vi "transfer char run_subvi_7_24_12a_PD.vi"(0 "VISA session":refnum<visa-resource-name>="GPIB0::17::INSTR", 5 "Var1 sweep settings":T4={"start"=40.0, "stop"=-40.0, "step (linear only)"=-1.0, "sweep spacing (linear: 0)"=0, "sweep mode"=FALSE, "compliance (V)"=100.0, "compliance (A)"=0.001} {"compliance (A)" format="%^.2e"; "compliance (V)" format="%.2f"; "sweep spacing (linear: 0)" items=["linear", "log 10", "log 25", "log 50"]; "step (linear only)" format="%.2f"; "stop" format="%.2f"; "start" format="%.2f"}, 7 "Var2 step settings":T3={"compliance (A)"=0.001, "compliance (V)"=100.0, "start"=-2.0, "total points"=2, "step"=-38.0} {"step" format="%.2f"; "start" format="%.2f"; "compliance (V)" format="%.2f"; "compliance (A)" format="%^.2e"}, 9 "integration time":u32(slide) scale=0.0..2.0, 11 "Input Path":path, 13 "Sample Properties:":T1 {"Date Created" format="%<%x>T"}) -> (1 "Trap Density-STS":dbl, 3 "Trap Density-VT":dbl, 4 "Mobility":dbl, 6 "graphic display":cluster{"trace":dbl[], "trace":dbl[]}(graph), 8 "On/Off Current":dbl, 10 "XY Graph":cluster{dbl[], "trace":dbl[]}[](graph), 12 "Vt":dbl, 14 "STS":dbl, 15 "error?":errorcluster)   [LabVIEW 2011]
uses:
  <vilib>/Utility/file.llb/Write To Spreadsheet File (DBL).vi
  <vilib>/Utility/file.llb/Read From Spreadsheet File (string).vi
  <vilib>/Utility/file.llb/Write To Spreadsheet File (string).vi
  <vilib>/Analysis/NI_AALPro.lvlib
panel:
  out "Array":string[][](array[string])
  in  "Output Path":path
  in  "Temp (K)":dbl=0.001 format="%^.2e"
  in  "NumPts":dbl=5.0
  out "Numeric":dbl
  out "Max R":i32[](listbox)
  out "min r":dbl
  out "max r":dbl
  out "error? 2":errorcluster
  in  "MAXIMUM":ext format="%.2e"
  in  "MINIMUM":ext=-1e-05 format="%_2e"
  out "graphic display 2":cluster{"trace":dbl[], "trace":dbl[]}(graph)
  in  "Y1 axis":string="Id"
  in  "Y2 axis settings":T2 {"MAXIMUM" format="%.9f"; "MINIMUM" format="%.9f"}
  in  "wait time parameter":dbl=1.0
  in  "Value (Either V or A) 4":dbl
  in  "Value (Either V or A) 3":dbl
  in  "Value (Either V or A) 2":dbl
  in  "Value (V or A)":dbl
  in  "compliance (A)":dbl=0.001 format="%^.2e"
  in  "compliance (V)":dbl=100.0 format="%^.2e"
  in  "Iname":string="Is"
  in  "Vname":string="Vs"
  in  "Function":u16(ring)=4 items=["disabled", "Var1", "Var2", "Var1'", "Constant"]
  in  "Mode":u16(ring)=4 items=["V", "I", "VPulse", "IPulse", "Common"]
  in  "Iname 4":string="I4"
  in  "Vname 4":string="V4"
  in  "Function 4":u16(ring)=4 items=["disabled", "Var1", "Var2", "Var1'", "Constant"]
  in  "Mode 4":u16(ring) items=["V", "I", "VPulse", "IPulse", "Common"]
  in  "Iname 3":string="Ig"
  in  "Vname 3":string="Vg"
  in  "Function 3":u16(ring)=1 items=["disabled", "Var1", "Var2", "Var1'", "Constant"]
  in  "Mode 3":u16(ring) items=["V", "I", "VPulse", "IPulse", "Common"]
  in  "Iname 2":string="Id"
  in  "Vname 2":string="Vd"
  in  "Function 2":u16(ring)=2 items=["disabled", "Var1", "Var2", "Var1'", "Constant"]
  in  "Mode 2":u16(ring) items=["V", "I", "VPulse", "IPulse", "Common"]
  in  "reset":bool=TRUE
  # "SMU1"
  # "SMU2"
  # "SMU3"
  # "SMU4"
  # "Sample Properties:"
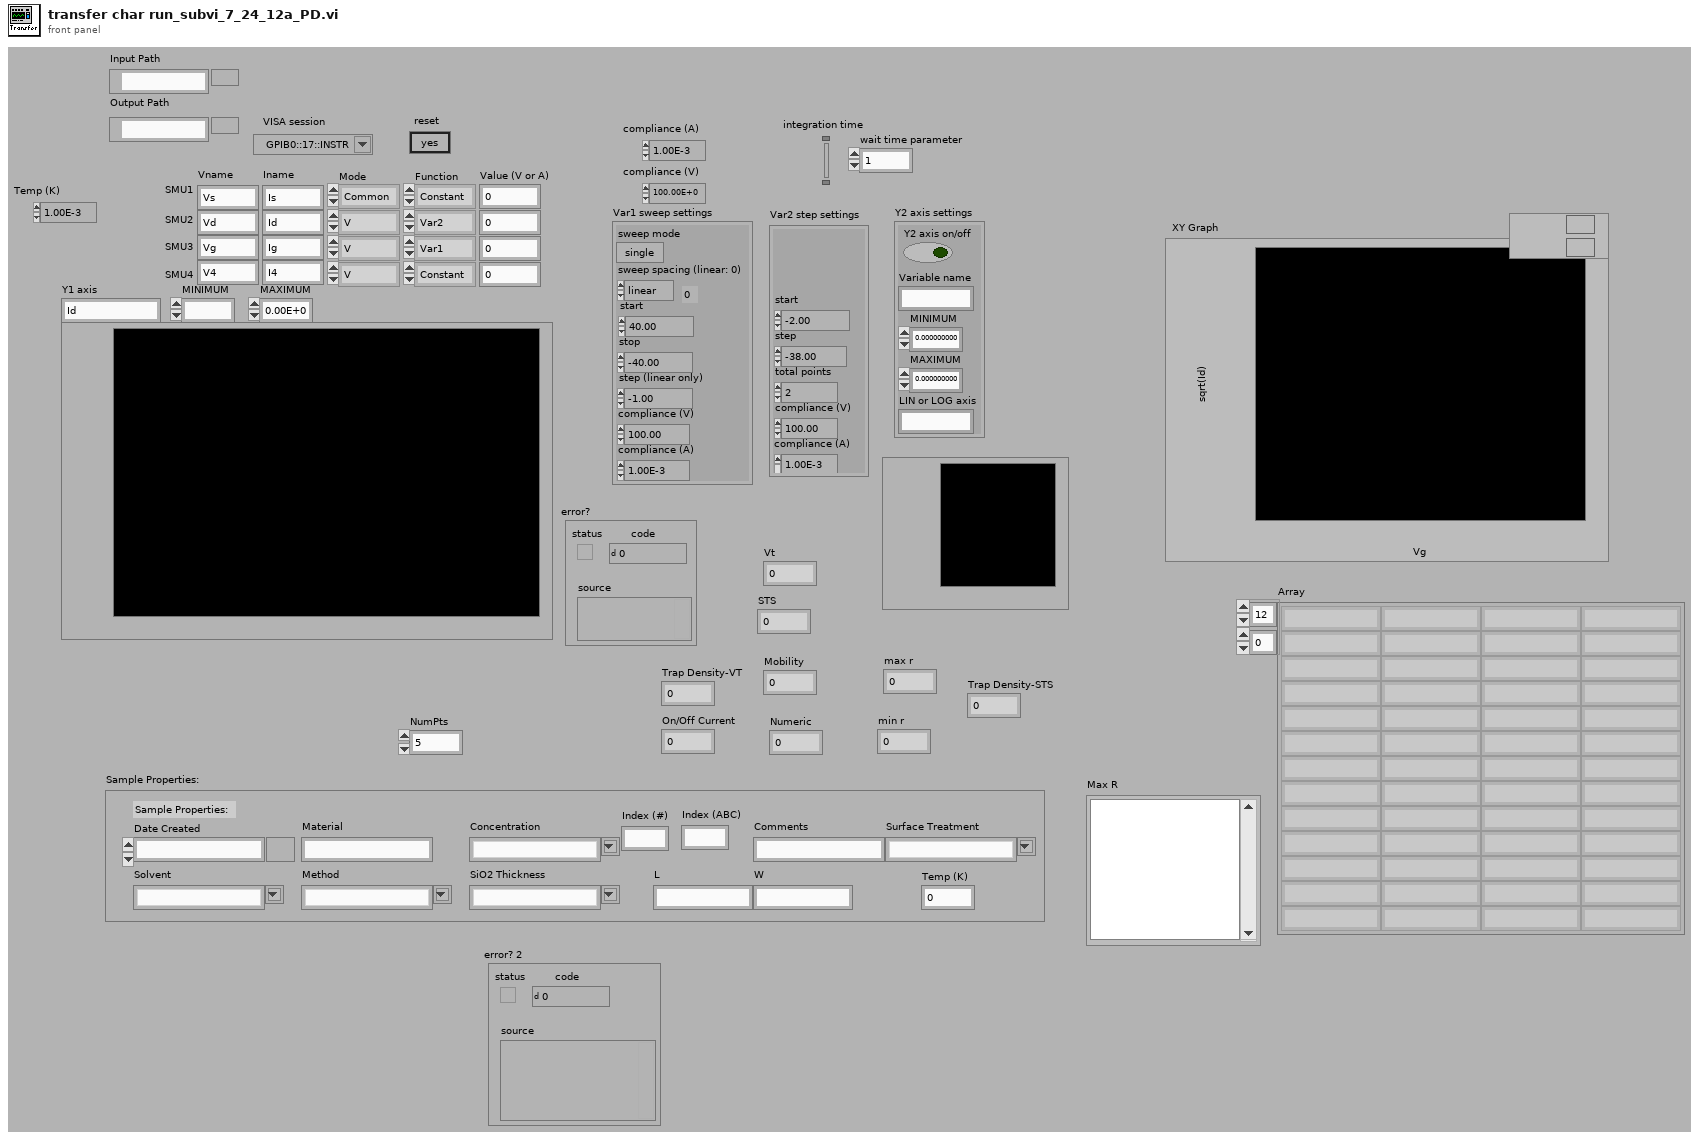
[diagram p1: front panel]
types:
  T1 = cluster{"Date Created":timestamp, "Material":string, "Solvent":string, "Concentration":string, "Method":string, "SiO2 Thickness":string, "Index (#)":string, "Index (ABC)":string, "L":string, "W":string, "Surface Treatment":string, "Comments":string, "Temp (K)":dbl}
  T2 = cluster{"Y2 axis on/off":bool, "MINIMUM":ext, "MAXIMUM":ext, "Variable name":string, "LIN or LOG axis":string}
  T3 = cluster{"compliance (A)":dbl, "compliance (V)":dbl, "start":dbl, "total points":u16, "step":dbl}
  T4 = cluster{"start":dbl, "stop":dbl, "step (linear only)":dbl, "sweep spacing (linear: 0)":u16, "sweep mode":bool, "compliance (V)":dbl, "compliance (A)":dbl}
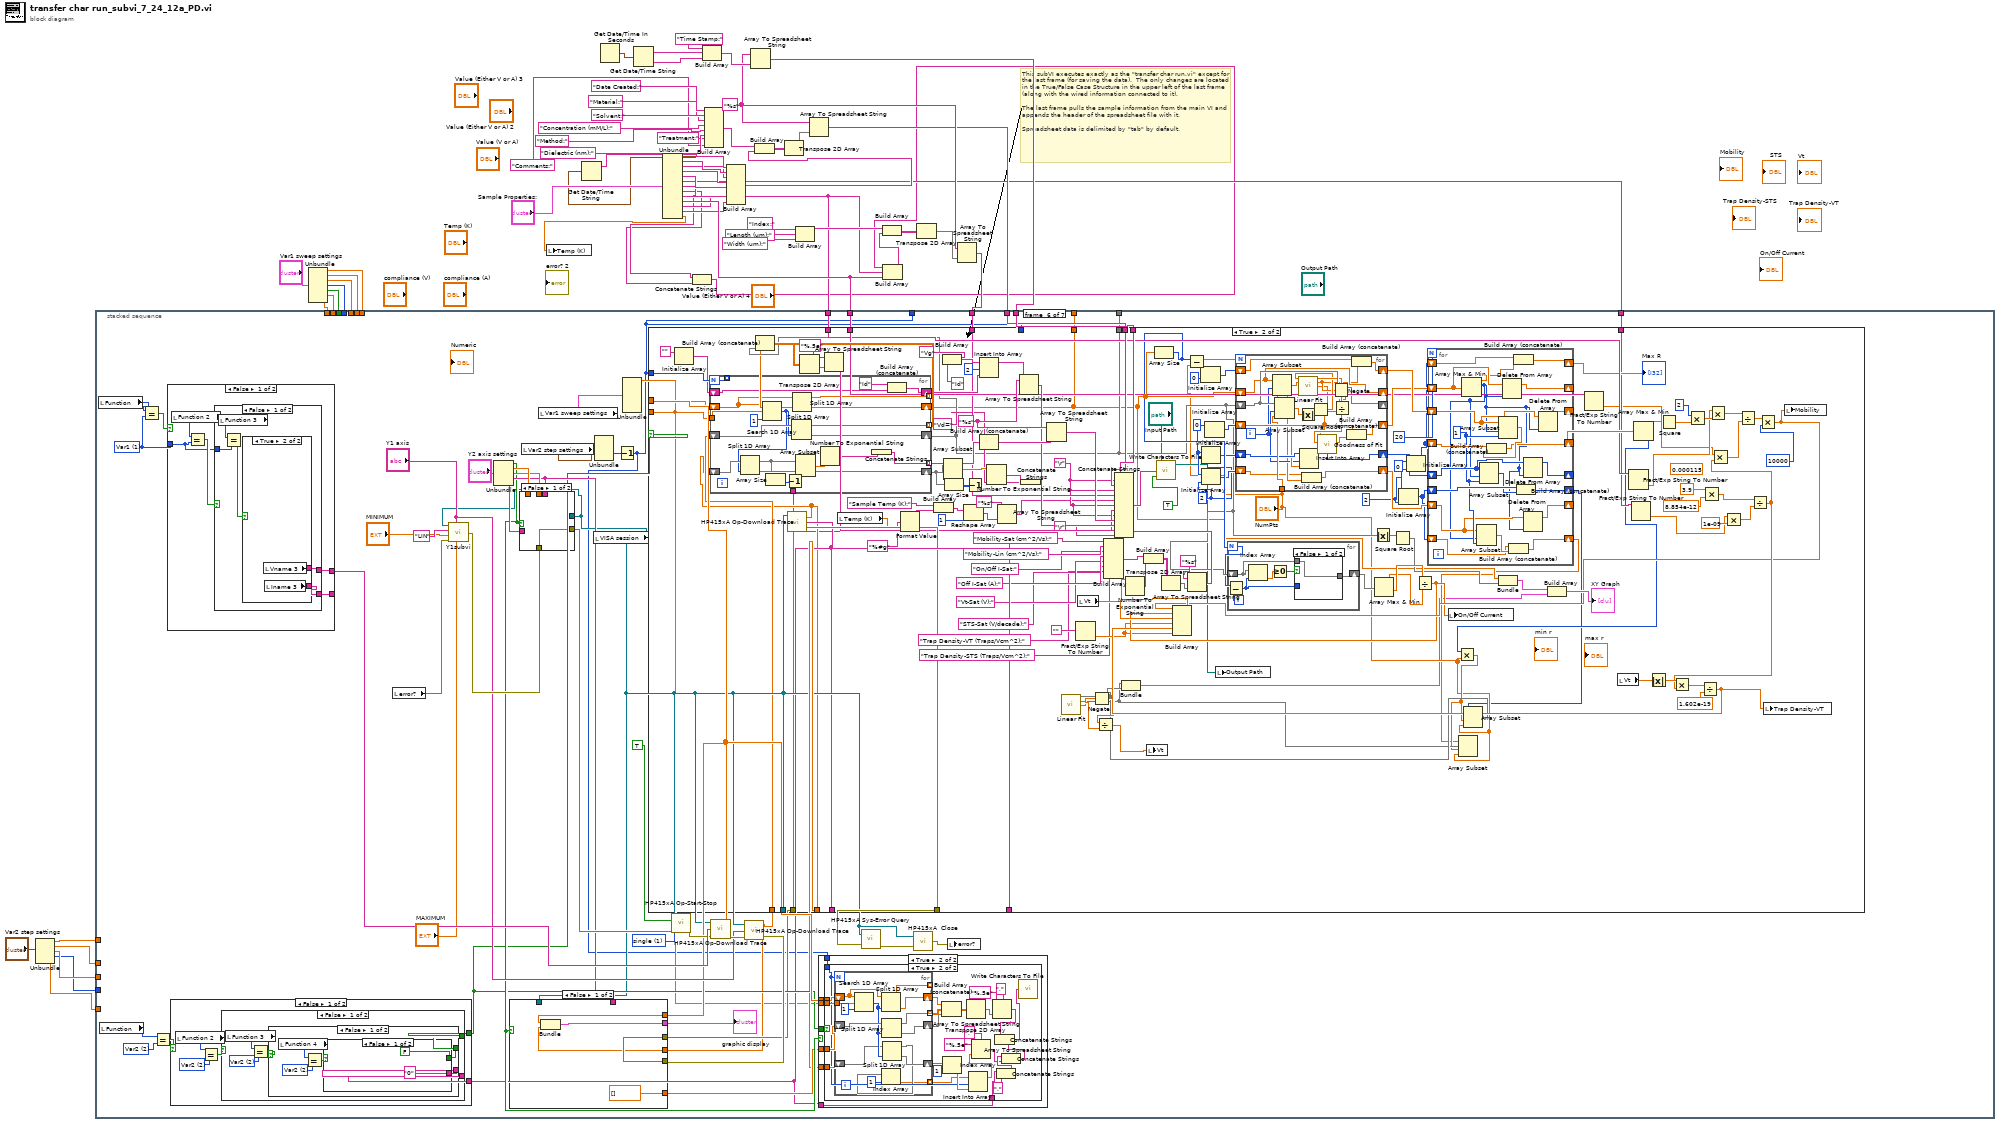
[diagram p0: block diagram]
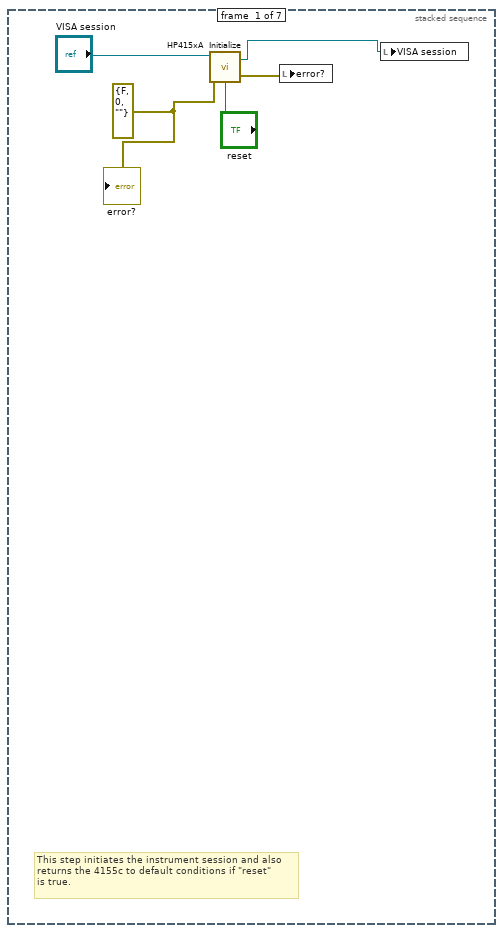
[diagram p2: hidden frame]
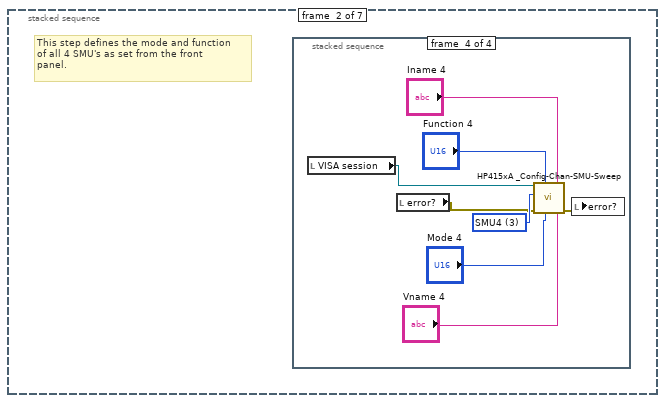
[diagram p3: hidden frame]
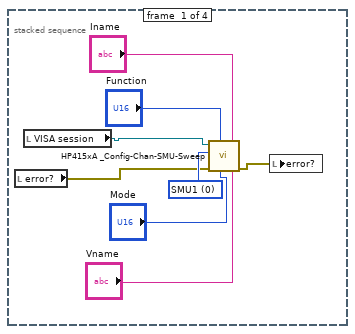
[diagram p4: hidden frame]
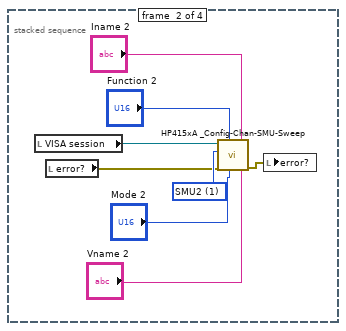
[diagram p5: hidden frame]
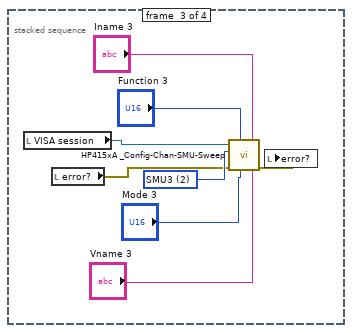
[diagram p6: hidden frame]
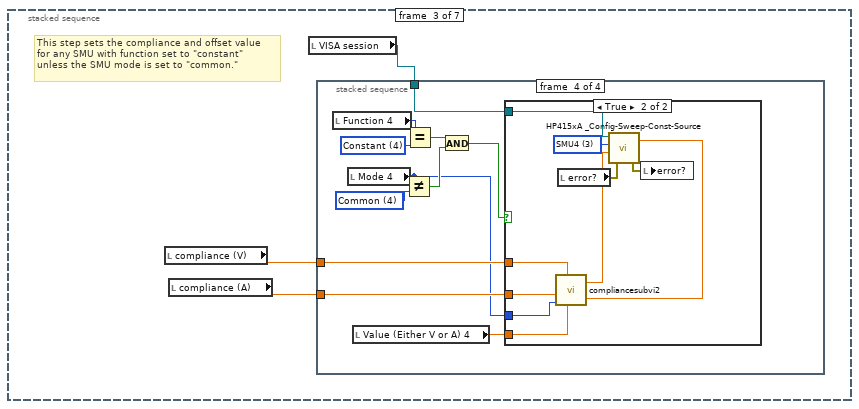
[diagram p7: hidden frame]
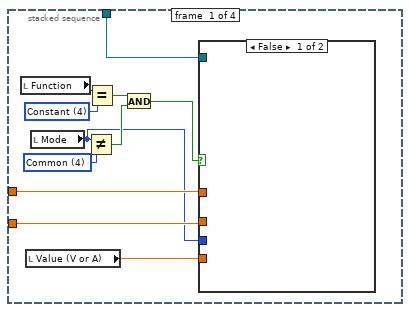
[diagram p8: hidden frame]
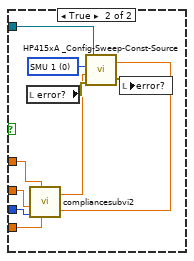
[diagram p9: hidden frame]
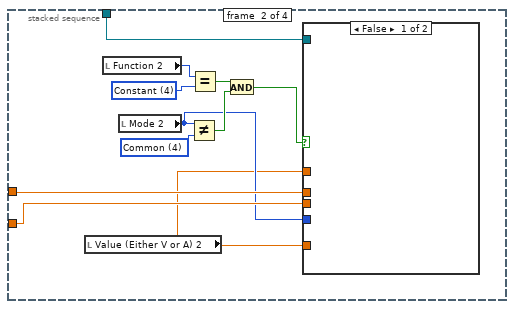
[diagram p10: hidden frame]
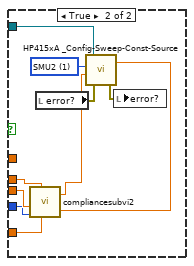
[diagram p11: hidden frame]
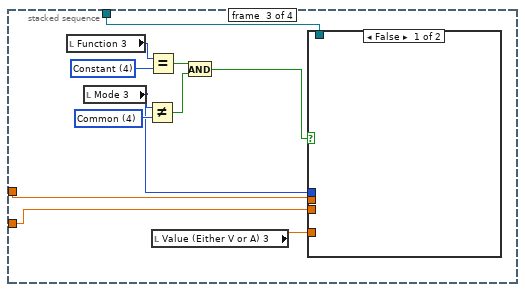
[diagram p12: hidden frame]
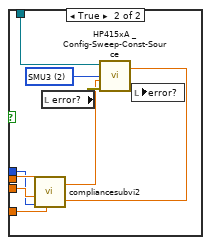
[diagram p13: hidden frame]
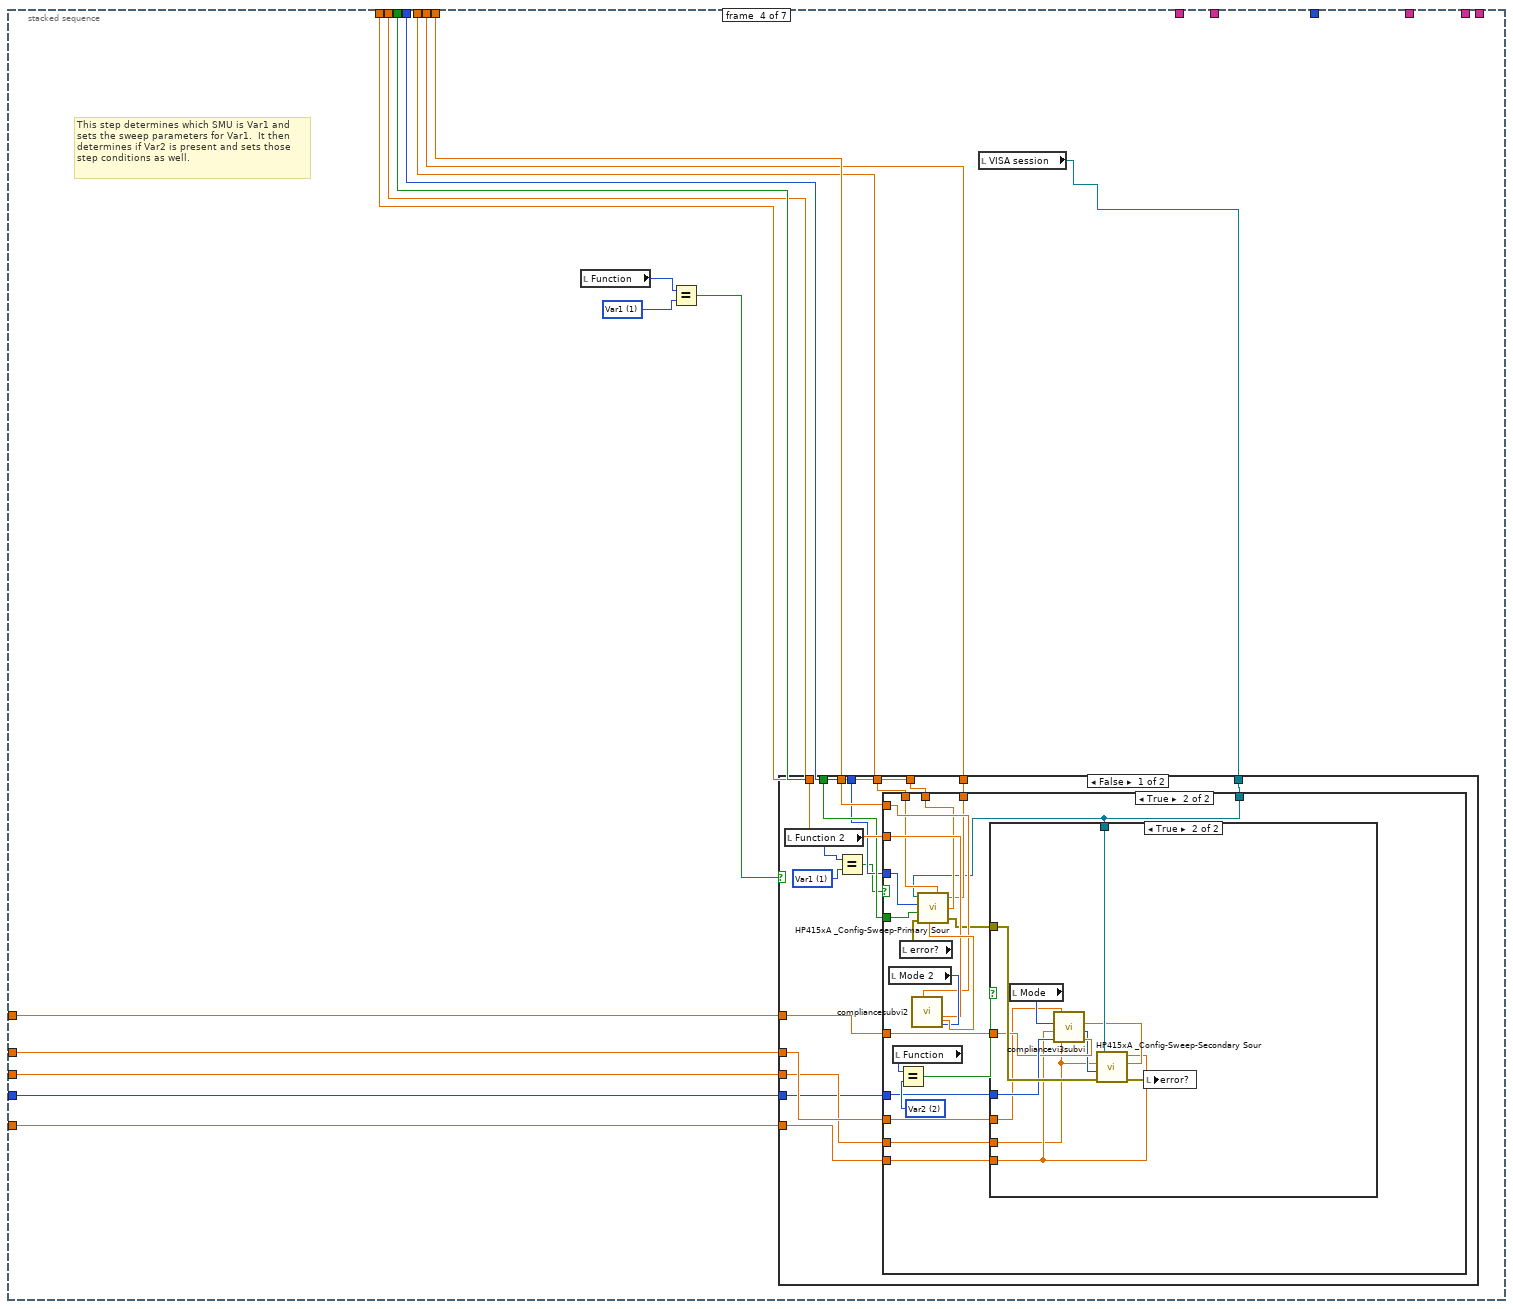
[diagram p15: hidden frame]
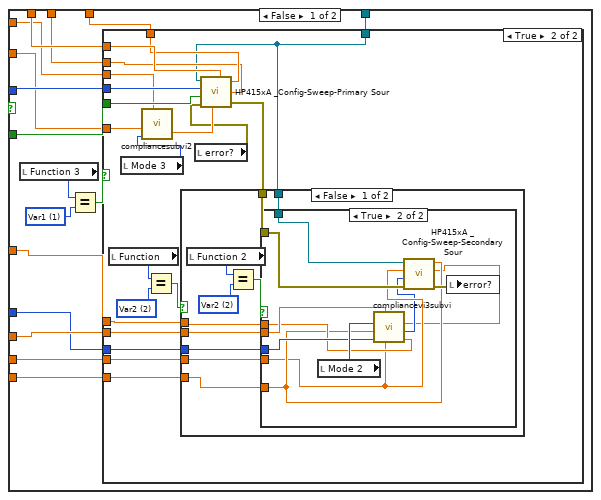
[diagram p16: hidden frame]
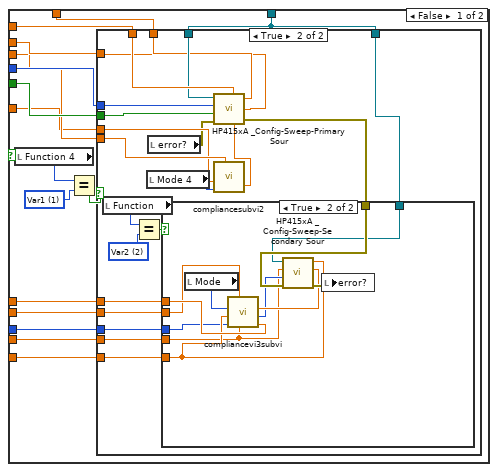
[diagram p17: hidden frame]
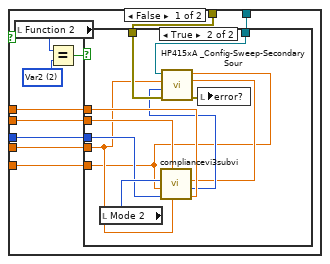
[diagram p19: hidden frame]
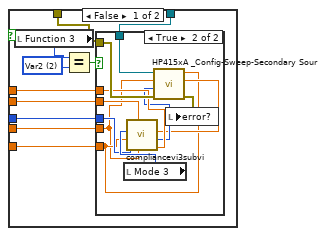
[diagram p20: hidden frame]
diagram:
  w31 = "%s"
  # "This subVI executes exactly as the \"transfer char run.vi\" except for the last frame (for saving the data).  The only changes are located in the True/False Case Structure in the upper left of the last frame (along with the wired information connected to it). \n\nThe last frame pulls the sample information from the main VI and appends the header of the spreadsheet file with it.\n\nSpreadsheet data is delimited by \"tab\" by default."
  n1 = Unbundle("Var2 step settings") -> ("compliance (A)"=w49:dbl, "compliance (V)"=w48:dbl, "start"=w47:dbl, "total points"=w46:u16, "step"=w45:dbl)
  n2 = Unbundle("Var1 sweep settings") -> ("start"=w57:dbl, "stop"=w56:dbl, "step (linear only)"=w55:dbl, "sweep spacing (linear: 0)"=w54:u16, "sweep mode"=w53:bool, "compliance (V)"=w52:dbl, "compliance (A)"=w51:dbl)
  n3 = Get Date/Time In Seconds() -> (seconds since 1Jan1904=w38:timestamp)
  n4 = Get Date/Time String(seconds (now)=w38) -> (date string=w37:string, time string=w36:string)  [unwired: 2 in]
  n5 = Unbundle("Sample Properties:") -> ("Date Created"=w16:timestamp, "Material"=w15:string, "Solvent"=w11:string, "Concentration"=w10:string, "Method"=w14:string, "SiO2 Thickness"=w9:string, "Index (#)"=w4:string, "Index (ABC)"=w3:string, "L"=w7:string, "W"=w8:string, "Surface Treatment"=w6:string, "Comments"=w5:string, "Temp (K)"=w1:dbl)
  n6 = local write "Temp (K)"(w1) -> ()
  n7 = Get Date/Time String(seconds (now)=w16) -> (date string=w43:string)  [unwired: 2 in, 1 out]
  n8 = Concatenate Strings(w4, w3) -> (w2:string)
  n9 = Build Array("Time Stamp:", w37, w36) -> (w35:string[])
  n10 = Build Array("Date Created:", "Material:", "Solvent:", "Concentration (mM/L):", "Method:", "Dielectric (nm):", "Treatment:", "Comments:") -> (w26:string[])
  n11 = Build Array(w43, w15, w11, w10, w14, w9, w6, w5) -> (w25:string[])
  n12 = Array To Spreadsheet String(array=w35, 3:w31) -> (spreadsheet string=w27:string)  [unwired: 1 in]
  n13 = Build Array(w26, w25) -> (w24:string[][])
  n14 = Transpose 2D Array(2D array=w24) -> (transposed array=w23:string[][])
  n15 = Build Array("Index:", "Length (um):", "Width (um):") -> (w22:string[])
  n16 = Array To Spreadsheet String(array=w23, 3:w31) -> (spreadsheet string=w30:string)  [unwired: 1 in]
  n17 = Build Array(w2, w7, w8) -> (w21:string[])
  n18 = Build Array(w22, w21) -> (w20:string[][])
  n19 = Transpose 2D Array(2D array=w20) -> (transposed array=w19:string[][])
  n20 = Array To Spreadsheet String(array=w19, 3:w31) -> (spreadsheet string=w18:string)  [unwired: 1 in]
  n21 = stacked-sequence {
    tunnel: w57 -> [_ _ _ w194 _ _ _]
    tunnel: w56 -> [_ _ _ w193 _ _ _]
    tunnel: w55 -> [_ _ _ w192 _ _ _]
    tunnel: w54 -> [_ _ _ w191 _ _ _]
    tunnel: w53 -> [_ _ _ w190 _ _ _]
    tunnel: w52 -> [_ _ _ w189 _ _ _]
    tunnel: w51 -> [_ _ _ w188 _ _ _]
    tunnel: w49 -> [_ _ _ w187 _ _ _]
    tunnel: w48 -> [_ _ _ w186 _ _ _]
    tunnel: w47 -> [_ _ _ w185 _ _ _]
    tunnel: w46 -> [_ _ _ w184 _ _ _]
    tunnel: w45 -> [_ _ _ w183 _ _ _]
    tunnel: w27 -> [_ _ _ _ _ w557 _]
    tunnel: w30 -> [_ _ _ _ _ w556 _]
    tunnel: w18 -> [_ _ _ _ _ w555 _]
    tunnel: [_ _ _ _ _ w554 _] -> _
    tunnel: [_ _ _ _ _ w553 _] -> _
    tunnel: [_ _ _ _ _ w550 _] -> _
    tunnel: w8 -> [_ _ _ _ _ w552 _]
    tunnel: w7 -> [_ _ _ _ _ w551 _]
    tunnel: w9 -> [_ _ _ _ _ w549 _]
    frame #0 {
      w62 = errorcluster {"status"=FALSE, "code"=0, "source"=""} ("error out")
      # "This step initiates the instrument session and also\nreturns the 4155c to default conditions if \"reset\"\nis true."
      n22 = call "HP415xA  Initialize.vi"("instrument descriptor"="VISA session", "reset"="reset", "error in (no error)"=w62) -> ("VISA session"=w59:refnum<visa-resource-name>, "error out"=w61:errorcluster)  [unwired: 2 in]
      n23 = local write "error?"(w61) -> ()
      n24 = local write "VISA session"(w59) -> ()
      "error?" <- w62
    }
    frame #1 {
      # "This step defines the mode and function\nof all 4 SMU's as set from the front\npanel."
      n25 = stacked-sequence {
        frame #0 {
          w71 = u32 0 items=["SMU1  ", "SMU2  ", "SMU3  ", "SMU4  ", "SMU5  ", "SMU6  "] ("unit to configure")
          n26 = local read "error?"() -> (w66:errorcluster)
          n27 = local read "VISA session"() -> (w64:refnum<visa-resource-name>)
          n28 = call "HP415xA _Config-Chan-SMU-Sweep.vi"("V name (max 6 chars)"="Vname", "I name (max 6 chars)"="Iname", "mode"="Mode", "function"="Function", "error in (no error)"=w66, "unit to configure"=w71, "VISA session"=w64) -> ("error out"=w65:errorcluster)  [unwired: 2 in]
          n29 = local write "error?"(w65) -> ()
        }
        frame #1 {
          w75 = u32 1 items=["SMU1  ", "SMU2  ", "SMU3  ", "SMU4  ", "SMU5  ", "SMU6  "] ("unit to configure")
          n30 = local read "VISA session"() -> (w72:refnum<visa-resource-name>)
          n31 = local read "error?"() -> (w73:errorcluster)
          n32 = call "HP415xA _Config-Chan-SMU-Sweep.vi"("V name (max 6 chars)"="Vname 2", "I name (max 6 chars)"="Iname 2", "mode"="Mode 2", "function"="Function 2", "error in (no error)"=w73, "unit to configure"=w75, "VISA session"=w72) -> ("error out"=w74:errorcluster)  [unwired: 2 in]
          n33 = local write "error?"(w74) -> ()
        }
        frame #2 {
          w83 = u32 2 items=["SMU1  ", "SMU2  ", "SMU3  ", "SMU4  ", "SMU5  ", "SMU6  "] ("unit to configure")
          n34 = local read "VISA session"() -> (w80:refnum<visa-resource-name>)
          n35 = local read "error?"() -> (w81:errorcluster)
          n36 = call "HP415xA _Config-Chan-SMU-Sweep.vi"("V name (max 6 chars)"="Vname 3", "I name (max 6 chars)"="Iname 3", "mode"="Mode 3", "function"="Function 3", "error in (no error)"=w81, "unit to configure"=w83, "VISA session"=w80) -> ("error out"=w82:errorcluster)  [unwired: 2 in]
          n37 = local write "error?"(w82) -> ()
        }
        frame #3 {
          w91 = u32 3 items=["SMU1  ", "SMU2  ", "SMU3  ", "SMU4  ", "SMU5  ", "SMU6  "] ("unit to configure")
          n38 = local read "VISA session"() -> (w88:refnum<visa-resource-name>)
          n39 = local read "error?"() -> (w90:errorcluster)
          n40 = call "HP415xA _Config-Chan-SMU-Sweep.vi"("V name (max 6 chars)"="Vname 4", "I name (max 6 chars)"="Iname 4", "mode"="Mode 4", "function"="Function 4", "error in (no error)"=w90, "unit to configure"=w91, "VISA session"=w88) -> ("error out"=w89:errorcluster)  [unwired: 2 in]
          n41 = local write "error?"(w89) -> ()
        }
      }
    }
    frame #2 {
      # "This step sets the compliance and offset value\nfor any SMU with function set to \"constant\"\nunless the SMU mode is set to \"common.\""
      n42 = local read "compliance (V)"() -> (w97:dbl)
      n43 = local read "compliance (A)"() -> (w98:dbl)
      n44 = local read "VISA session"() -> (w96:refnum<visa-resource-name>)
      n45 = stacked-sequence {
        tunnel: w96 -> [w107 w127 w146 w166]
        tunnel: w98 -> [w101 w123 w144 w164]
        tunnel: w97 -> [w100 w122 w143 w165]
        frame #0 {
          w105 = u16 4 items=["V", "I", "VPulse", "IPulse", "Common"] ("Mode")
          w109 = u16 4 items=["disabled", "Var1", "Var2", "Var1'", "Constant"] ("Function")
          n46 = local read "Function"() -> (w108:u16)
          n47 = local read "Value (V or A)"() -> (w102:dbl)
          n48 = local read "Mode"() -> (w99:u16)
          n49 = Not Equal?(x=w99, y=w105) -> (x != y?=w104:bool)
          n50 = Equal?(x=w108, y=w109) -> (x = y?=w106:bool)
          n51 = And(x=w106, y=w104) -> (x .and. y?=w103:bool)
          n52 = case shown="False" w103 {
            tunnel: w107 -> [_ w119]
            tunnel: w100 -> [_ w115]
            tunnel: w101 -> [_ w114]
            tunnel: w102 -> [_ w111]
            tunnel: w99 -> [_ w112]
            frame False {
            }
            frame True {
              w118 = u16 0 items=["SMU 1", "SMU2", "SMU3", "SMU4", "SMU5", "SMU6", "VSU1", "VSU2"] ("unit (SMU1:0)")
              n53 = local read "error?"() -> (w117:errorcluster)
              n54 = call "compliancesubvi2.vi"("Value1"=w111, "compliance (V)"=w115, "Mode"=w112, "compliance (A)"=w114) -> ("compliance"=w113:dbl, "constant"=w110:dbl)  [unwired: 2 in]
              n55 = call "HP415xA _Config-Sweep-Const-Source.vi"("compliance (SMUs only)"=w113, "error in (no error)"=w117, "source (V or A)"=w110, "unit (SMU1:0)"=w118, "VISA session"=w119) -> ("error out"=w116:errorcluster)
              n56 = local write "error?"(w116) -> ()
            }
          }
        }
        frame #1 {
          w124 = u16 4 items=["V", "I", "VPulse", "IPulse", "Common"] ("Mode 2")
          w125 = u16 4 items=["disabled", "Var1", "Var2", "Var1'", "Constant"] ("Function 2")
          n57 = local read "Value (Either V or A) 2"() -> (w120:dbl)
          n58 = local read "Function 2"() -> (w126:u16)
          n59 = local read "Mode 2"() -> (w121:u16)
          n60 = Not Equal?(x=w121, y=w124) -> (x != y?=w129:bool)
          n61 = Equal?(x=w126, y=w125) -> (x = y?=w130:bool)
          n62 = And(x=w130, y=w129) -> (x .and. y?=w128:bool)
          n63 = case shown="False" w128 {
            tunnel: w127 -> [_ w140]
            tunnel: w122 -> [_ w138]
            tunnel: w123 -> [_ w137]
            tunnel: w120 -> [_ _]
            tunnel: w121 -> [_ w133]
            tunnel: w120 -> [_ w132]
            frame False {
            }
            frame True {
              w139 = u16 1 items=["SMU 1", "SMU2", "SMU3", "SMU4", "SMU5", "SMU6", "VSU1", "VSU2"] ("unit (SMU1:0)")
              n64 = call "compliancesubvi2.vi"("Value1"=w132, "compliance (V)"=w138, "Mode"=w133, "compliance (A)"=w137) -> ("compliance"=w136:dbl, "constant"=w131:dbl)  [unwired: 2 in]
              n65 = local read "error?"() -> (w135:errorcluster)
              n66 = call "HP415xA _Config-Sweep-Const-Source.vi"("compliance (SMUs only)"=w136, "error in (no error)"=w135, "source (V or A)"=w131, "unit (SMU1:0)"=w139, "VISA session"=w140) -> ("error out"=w134:errorcluster)
              n67 = local write "error?"(w134) -> ()
            }
          }
        }
        frame #2 {
          w148 = u16 4 items=["V", "I", "VPulse", "IPulse", "Common"] ("Mode 2")
          w149 = u16 4 items=["disabled", "Var1", "Var2", "Var1'", "Constant"] ("Function 2")
          n68 = local read "Function 3"() -> (w147:u16)
          n69 = local read "Mode 3"() -> (w142:u16)
          n70 = Not Equal?(x=w142, y=w148) -> (x != y?=w150:bool)
          n71 = Equal?(x=w147, y=w149) -> (x = y?=w151:bool)
          n72 = local read "Value (Either V or A) 3"() -> (w145:dbl)
          n73 = And(x=w151, y=w150) -> (x .and. y?=w141:bool)
          n74 = case shown="False" w141 {
            tunnel: w146 -> [_ w159]
            tunnel: w145 -> [_ w153]
            tunnel: w144 -> [_ w156]
            tunnel: w143 -> [_ w155]
            tunnel: w142 -> [_ w154]
            frame False {
            }
            frame True {
              w158 = u16 2 items=["SMU 1", "SMU2", "SMU3", "SMU4", "SMU5", "SMU6", "VSU1", "VSU2"] ("unit (SMU1:0)")
              n75 = call "compliancesubvi2.vi"("Value1"=w153, "compliance (V)"=w155, "Mode"=w154, "compliance (A)"=w156) -> ("compliance"=w157:dbl, "constant"=w152:dbl)  [unwired: 2 in]
              n76 = local read "error?"() -> (w161:errorcluster)
              n77 = call "HP415xA _Config-Sweep-Const-Source.vi"("compliance (SMUs only)"=w157, "error in (no error)"=w161, "source (V or A)"=w152, "unit (SMU1:0)"=w158, "VISA session"=w159) -> ("error out"=w160:errorcluster)
              n78 = local write "error?"(w160) -> ()
            }
          }
        }
        frame #3 {
          w168 = u16 4 items=["V", "I", "VPulse", "IPulse", "Common"] ("Mode 4")
          w169 = u16 4 items=["disabled", "Var1", "Var2", "Var1'", "Constant"] ("Function 4")
          n79 = local read "Function 4"() -> (w170:u16)
          n80 = local read "Mode 4"() -> (w163:u16)
          n81 = local read "Value (Either V or A) 4"() -> (w162:dbl)
          n82 = Not Equal?(x=w163, y=w168) -> (x != y?=w171:bool)
          n83 = Equal?(x=w170, y=w169) -> (x = y?=w172:bool)
          n84 = And(x=w172, y=w171) -> (x .and. y?=w167:bool)
          n85 = case shown="True" w167 {
            tunnel: w166 -> [_ w181]
            tunnel: w165 -> [_ w177]
            tunnel: w164 -> [_ w178]
            tunnel: w163 -> [_ w176]
            tunnel: w162 -> [_ w175]
            frame False {
            }
            frame True {
              w182 = u16 3 items=["SMU 1", "SMU2", "SMU3", "SMU4", "SMU5", "SMU6", "VSU1", "VSU2"] ("unit (SMU1:0)")
              n86 = call "compliancesubvi2.vi"("Value1"=w175, "compliance (V)"=w177, "Mode"=w176, "compliance (A)"=w178) -> ("compliance"=w174:dbl, "constant"=w173:dbl)  [unwired: 2 in]
              n87 = local read "error?"() -> (w180:errorcluster)
              n88 = call "HP415xA _Config-Sweep-Const-Source.vi"("compliance (SMUs only)"=w174, "error in (no error)"=w180, "source (V or A)"=w173, "unit (SMU1:0)"=w182, "VISA session"=w181) -> ("error out"=w179:errorcluster)
              n89 = local write "error?"(w179) -> ()
            }
          }
        }
      }
    }
    frame #3 {
      w198 = u16 1 items=["disabled", "Var1", "Var2", "Var1'", "Constant"] ("Function")
      # "This step determines which SMU is Var1 and\nsets the sweep parameters for Var1.  It then\ndetermines if Var2 is present and sets those\nstep conditions as well."
      n90 = local read "Function"() -> (w197:u16)
      n91 = Equal?(x=w197, y=w198) -> (x = y?=w196:bool)
      n92 = local read "VISA session"() -> (w195:refnum<visa-resource-name>)
      n93 = case shown="False" w196 {
        tunnel: w189 -> [w211 w487]
        tunnel: w188 -> [w212 w486]
        tunnel: w191 -> [w209 w485]
        tunnel: w190 -> [w210 w484]
        tunnel: w192 -> [w206 w483]
        tunnel: w193 -> [w205 w482]
        tunnel: w194 -> [w207 w481]
        tunnel: w195 -> [w208 w470]
        tunnel: w187 -> [w203 w476]
        tunnel: w186 -> [w202 w475]
        tunnel: w185 -> [w201 w474]
        tunnel: w184 -> [w200 w473]
        tunnel: w183 -> [w199 w472]
        frame False {
          w214 = u16 1 items=["disabled", "Var1", "Var2", "Var1'", "Constant"] ("Function")
          n94 = local read "Function 2"() -> (w213:u16)
          n95 = Equal?(x=w213, y=w214) -> (x = y?=w204:bool)
          n96 = case shown="True" w204 {
            tunnel: w212 -> [w220 w413]
            tunnel: w211 -> [w221 w412]
            tunnel: w210 -> [w222 w411]
            tunnel: w209 -> [w223 w410]
            tunnel: w208 -> [w227 w399]
            tunnel: w207 -> [w226 w409]
            tunnel: w206 -> [w224 w408]
            tunnel: w205 -> [w225 w407]
            tunnel: w203 -> [w219 w402]
            tunnel: w202 -> [w218 w401]
            tunnel: w201 -> [w216 w400]
            tunnel: w200 -> [w217 w397]
            tunnel: w199 -> [w215 w396]
            frame False {
              w230 = u16 1 items=["disabled", "Var1", "Var2", "Var1'", "Constant"] ("Function")
              n97 = local read "Function 3"() -> (w229:u16)
              n98 = Equal?(x=w229, y=w230) -> (x = y?=w228:bool)
              n99 = case shown="True" w228 {
                tunnel: w227 -> [w231 w324]
                tunnel: w226 -> [w243 w341]
                tunnel: w225 -> [w240 w340]
                tunnel: w224 -> [w239 w339]
                tunnel: w223 -> [w242 w338]
                tunnel: w222 -> [w241 w337]
                tunnel: w221 -> [w238 w336]
                tunnel: w220 -> [w237 w335]
                tunnel: w219 -> [w236 w328]
                tunnel: w218 -> [w235 w327]
                tunnel: w217 -> [w234 w326]
                tunnel: w216 -> [w233 w323]
                tunnel: w215 -> [w232 w322]
                frame False {
                  w246 = u16 1 items=["disabled", "Var1", "Var2", "Var1'", "Constant"] ("Function")
                  n100 = local read "Function 4"() -> (w245:u16)
                  n101 = Equal?(x=w245, y=w246) -> (x = y?=w244:bool)
                  n102 = case shown="True" w244 {
                    tunnel: w243 -> [_ w265]
                    tunnel: w231 -> [_ w264]
                    tunnel: w242 -> [_ w263]
                    tunnel: w241 -> [_ w262]
                    tunnel: w240 -> [_ w261]
                    tunnel: w239 -> [_ w260]
                    tunnel: w238 -> [_ w259]
                    tunnel: w237 -> [_ w258]
                    tunnel: w236 -> [_ w253]
                    tunnel: w235 -> [_ w252]
                    tunnel: w234 -> [_ w251]
                    tunnel: w233 -> [_ w250]
                    tunnel: w232 -> [_ w249]
                    tunnel: w231 -> [_ w247]
                    frame False {
                    }
                    frame True {
                      w256 = u16 2 items=["disabled", "Var1", "Var2", "Var1'", "Constant"] ("Function")
                      n103 = local read "Function"() -> (w255:u16)
                      n104 = Equal?(x=w255, y=w256) -> (x = y?=w254:bool)
                      n105 = local read "Mode 4"() -> (w267:u16)
                      n106 = local read "error?"() -> (w257:errorcluster)
                      n107 = call "compliancesubvi2.vi"("compliance (V)"=w259, "Mode"=w267, "compliance (A)"=w258) -> ("compliance"=w266:dbl)  [unwired: 3 in, 1 out]
                      n108 = call "HP415xA _Config-Sweep-Primary Sour.vi"("step (linear only)"=w260, "stop"=w261, "start"=w265, "compliance"=w266, "error in (no error)"=w257, "sweep mode"=w262, "sweep spacing (linear: 0)"=w263, "VISA session"=w264) -> ("error out"=w248:errorcluster)  [unwired: 2 in]
                      n109 = case shown="True" w254 {
                        tunnel: w253 -> [w274 w317]
                        tunnel: w252 -> [w273 w312]
                        tunnel: w251 -> [w272 w311]
                        tunnel: w250 -> [w271 w313]
                        tunnel: w249 -> [w270 w316]
                        tunnel: w248 -> [w269 w319]
                        tunnel: w247 -> [w268 w318]
                        frame False {
                          w277 = u16 2 items=["disabled", "Var1", "Var2", "Var1'", "Constant"] ("Function")
                          n110 = local read "Function 2"() -> (w276:u16)
                          n111 = Equal?(x=w276, y=w277) -> (x = y?=w275:bool)
                          n112 = case shown="True" w275 {
                            tunnel: w274 -> [w285 w305]
                            tunnel: w273 -> [w284 w306]
                            tunnel: w272 -> [w283 w304]
                            tunnel: w271 -> [w282 w302]
                            tunnel: w270 -> [w281 w300]
                            tunnel: w269 -> [w280 w310]
                            tunnel: w268 -> [w278 w309]
                            frame False {
                              w287 = u16 2 items=["disabled", "Var1", "Var2", "Var1'", "Constant"] ("Function")
                              n113 = local read "Function 3"() -> (w279:u16)
                              n114 = Equal?(x=w279, y=w287) -> (x = y?=w286:bool)
                              n115 = case shown="True" w286 {
                                tunnel: w285 -> [_ w293]
                                tunnel: w284 -> [_ w294]
                                tunnel: w283 -> [_ w295]
                                tunnel: w282 -> [_ w289]
                                tunnel: w281 -> [_ w290]
                                tunnel: w280 -> [w288 w299]
                                tunnel: w278 -> [_ w298]
                                frame False {
                                n116 = local write "error?"(w288) -> ()
                                }
                                frame True {
                                n117 = local read "Mode 3"() -> (w297:u16)
                                n118 = call "compliancevi3subvi.vi"("compliance (A)"=w293, "start"=w289, "compliance (V)"=w294, "total points"=w295, "step"=w290, "Mode"=w297) -> ("total points 2"=w292:u16, "compliance"=w291:dbl)  [unwired: 1 in, 1 out]
                                n119 = call "HP415xA _Config-Sweep-Secondary Sour.vi"("compliance"=w291, "step"=w290, "error in (no error)"=w299, "total points"=w292, "start"=w289, "VISA session"=w298) -> ("error out"=w296:errorcluster)  [unwired: 1 in]
                                n120 = local write "error?"(w296) -> ()
                                }
                              }
                            }
                            frame True {
                              n121 = local read "Mode 2"() -> (w308:u16)
                              n122 = call "compliancevi3subvi.vi"("compliance (A)"=w305, "start"=w302, "compliance (V)"=w306, "total points"=w304, "step"=w300, "Mode"=w308) -> ("total points 2"=w303:u16, "compliance"=w301:dbl)  [unwired: 1 in, 1 out]
                              n123 = call "HP415xA _Config-Sweep-Secondary Sour.vi"("compliance"=w301, "step"=w300, "error in (no error)"=w310, "total points"=w303, "start"=w302, "VISA session"=w309) -> ("error out"=w307:errorcluster)  [unwired: 1 in]
                              n124 = local write "error?"(w307) -> ()
                            }
                          }
                        }
                        frame True {
                          n125 = local read "Mode"() -> (w321:u16)
                          n126 = call "compliancevi3subvi.vi"("compliance (A)"=w317, "start"=w313, "compliance (V)"=w312, "total points"=w311, "step"=w316, "Mode"=w321) -> ("total points 2"=w314:u16, "compliance"=w315:dbl)  [unwired: 1 in, 1 out]
                          n127 = call "HP415xA _Config-Sweep-Secondary Sour.vi"("compliance"=w315, "step"=w316, "error in (no error)"=w319, "total points"=w314, "start"=w313, "VISA session"=w318) -> ("error out"=w320:errorcluster)  [unwired: 1 in]
                          n128 = local write "error?"(w320) -> ()
                        }
                      }
                    }
                  }
                }
                frame True {
                  w331 = u16 2 items=["disabled", "Var1", "Var2", "Var1'", "Constant"] ("Function")
                  n129 = local read "Function"() -> (w330:u16)
                  n130 = local read "Mode 3"() -> (w333:u16)
                  n131 = call "compliancesubvi2.vi"("compliance (V)"=w336, "Mode"=w333, "compliance (A)"=w335) -> ("compliance"=w334:dbl)  [unwired: 3 in, 1 out]
                  n132 = Equal?(x=w330, y=w331) -> (x = y?=w329:bool)
                  n133 = local read "error?"() -> (w332:errorcluster)
                  n134 = call "HP415xA _Config-Sweep-Primary Sour.vi"("step (linear only)"=w339, "stop"=w340, "start"=w341, "compliance"=w334, "error in (no error)"=w332, "sweep mode"=w337, "sweep spacing (linear: 0)"=w338, "VISA session"=w324) -> ("error out"=w325:errorcluster)  [unwired: 2 in]
                  n135 = case shown="False" w329 {
                    tunnel: w328 -> [w346 w391]
                    tunnel: w327 -> [w345 w390]
                    tunnel: w326 -> [w343 w389]
                    tunnel: w325 -> [w348 w394]
                    tunnel: w324 -> [w347 w393]
                    tunnel: w323 -> [w342 w386]
                    tunnel: w322 -> [w344 w385]
                    frame False {
                      w351 = u16 2 items=["disabled", "Var1", "Var2", "Var1'", "Constant"] ("Function")
                      n136 = local read "Function 2"() -> (w350:u16)
                      n137 = Equal?(x=w350, y=w351) -> (x = y?=w349:bool)
                      n138 = case shown="True" w349 {
                        tunnel: w348 -> [w358 w383]
                        tunnel: w347 -> [w357 w382]
                        tunnel: w346 -> [w356 w378]
                        tunnel: w345 -> [w355 w379]
                        tunnel: w344 -> [w352 w377]
                        tunnel: w343 -> [w354 w380]
                        tunnel: w342 -> [w353 w376]
                        frame False {
                          w361 = u16 2 items=["disabled", "Var1", "Var2", "Var1'", "Constant"] ("Function")
                          n139 = local read "Function 4"() -> (w360:u16)
                          n140 = Equal?(x=w360, y=w361) -> (x = y?=w359:bool)
                          n141 = case shown="True" w359 {
                            tunnel: w358 -> [w362 w371]
                            tunnel: w357 -> [_ w372]
                            tunnel: w356 -> [_ w368]
                            tunnel: w355 -> [_ w369]
                            tunnel: w354 -> [_ w367]
                            tunnel: w353 -> [_ w364]
                            tunnel: w352 -> [_ w363]
                            frame False {
                              n142 = local write "error?"(w362) -> ()
                            }
                            frame True {
                              n143 = local read "Mode 4"() -> (w373:u16)
                              n144 = call "compliancevi3subvi.vi"("compliance (A)"=w368, "start"=w364, "compliance (V)"=w369, "total points"=w367, "step"=w363, "Mode"=w373) -> ("total points 2"=w366:u16, "compliance"=w365:dbl)  [unwired: 1 in, 1 out]
                              n145 = call "HP415xA _Config-Sweep-Secondary Sour.vi"("compliance"=w365, "step"=w363, "error in (no error)"=w371, "total points"=w366, "start"=w364, "VISA session"=w372) -> ("error out"=w370:errorcluster)  [unwired: 1 in]
                              n146 = local write "error?"(w370) -> ()
                            }
                          }
                        }
                        frame True {
                          n147 = local read "Mode 2"() -> (w384:u16)
                          n148 = call "compliancevi3subvi.vi"("compliance (A)"=w378, "start"=w376, "compliance (V)"=w379, "total points"=w380, "step"=w377, "Mode"=w384) -> ("total points 2"=w375:u16, "compliance"=w374:dbl)  [unwired: 1 in, 1 out]
                          n149 = call "HP415xA _Config-Sweep-Secondary Sour.vi"("compliance"=w374, "step"=w377, "error in (no error)"=w383, "total points"=w375, "start"=w376, "VISA session"=w382) -> ("error out"=w381:errorcluster)  [unwired: 1 in]
                          n150 = local write "error?"(w381) -> ()
                        }
                      }
                    }
                    frame True {
                      n151 = local read "Mode"() -> (w395:u16)
                      n152 = call "compliancevi3subvi.vi"("compliance (A)"=w391, "start"=w386, "compliance (V)"=w390, "total points"=w389, "step"=w385, "Mode"=w395) -> ("total points 2"=w388:u16, "compliance"=w387:dbl)  [unwired: 1 in, 1 out]
                      n153 = call "HP415xA _Config-Sweep-Secondary Sour.vi"("compliance"=w387, "step"=w385, "error in (no error)"=w394, "total points"=w388, "start"=w386, "VISA session"=w393) -> ("error out"=w392:errorcluster)  [unwired: 1 in]
                      n154 = local write "error?"(w392) -> ()
                    }
                  }
                }
              }
            }
            frame True {
              w405 = u16 2 items=["disabled", "Var1", "Var2", "Var1'", "Constant"] ("Function")
              n155 = local read "Mode 2"() -> (w414:u16)
              n156 = local read "Function"() -> (w404:u16)
              n157 = Equal?(x=w404, y=w405) -> (x = y?=w403:bool)
              n158 = local read "error?"() -> (w406:errorcluster)
              n159 = call "compliancesubvi2.vi"("compliance (V)"=w412, "Mode"=w414, "compliance (A)"=w413) -> ("compliance"=w415:dbl)  [unwired: 3 in, 1 out]
              n160 = call "HP415xA _Config-Sweep-Primary Sour.vi"("step (linear only)"=w408, "stop"=w407, "start"=w409, "compliance"=w415, "error in (no error)"=w406, "sweep mode"=w411, "sweep spacing (linear: 0)"=w410, "VISA session"=w399) -> ("error out"=w398:errorcluster)  [unwired: 2 in]
              n161 = case shown="True" w403 {
                tunnel: w402 -> [w421 w464]
                tunnel: w401 -> [w420 w463]
                tunnel: w400 -> [w418 w459]
                tunnel: w399 -> [w423 w469]
                tunnel: w398 -> [w417 w468]
                tunnel: w397 -> [w419 w465]
                tunnel: w396 -> [w416 w461]
                frame False {
                  w425 = u16 2 items=["disabled", "Var1", "Var2", "Var1'", "Constant"] ("Function")
                  n162 = local read "Function 3"() -> (w424:u16)
                  n163 = Equal?(x=w424, y=w425) -> (x = y?=w422:bool)
                  n164 = case shown="True" w422 {
                    tunnel: w423 -> [w431 w457]
                    tunnel: w421 -> [w430 w454]
                    tunnel: w420 -> [w428 w452]
                    tunnel: w419 -> [w429 w453]
                    tunnel: w418 -> [w426 w450]
                    tunnel: w417 -> [w432 w456]
                    tunnel: w416 -> [w427 w448]
                    frame False {
                      w435 = u16 2 items=["disabled", "Var1", "Var2", "Var1'", "Constant"] ("Function")
                      n165 = local read "Function 4"() -> (w434:u16)
                      n166 = Equal?(x=w434, y=w435) -> (x = y?=w433:bool)
                      n167 = case shown="True" w433 {
                        tunnel: w432 -> [w436 w447]
                        tunnel: w431 -> [_ w446]
                        tunnel: w430 -> [_ w443]
                        tunnel: w429 -> [_ w444]
                        tunnel: w428 -> [_ w442]
                        tunnel: w427 -> [_ w438]
                        tunnel: w426 -> [_ w439]
                        frame False {
                          n168 = local write "error?"(w436) -> ()
                        }
                        frame True {
                          n169 = local read "Mode 4"() -> (w441:u16)
                          n170 = call "compliancevi3subvi.vi"("compliance (A)"=w443, "start"=w439, "compliance (V)"=w442, "total points"=w444, "step"=w438, "Mode"=w441) -> ("total points 2"=w440:u16, "compliance"=w437:dbl)  [unwired: 1 in, 1 out]
                          n171 = call "HP415xA _Config-Sweep-Secondary Sour.vi"("compliance"=w437, "step"=w438, "error in (no error)"=w447, "total points"=w440, "start"=w439, "VISA session"=w446) -> ("error out"=w445:errorcluster)  [unwired: 1 in]
                          n172 = local write "error?"(w445) -> ()
                        }
                      }
                    }
                    frame True {
                      n173 = local read "Mode 3"() -> (w458:u16)
                      n174 = call "compliancevi3subvi.vi"("compliance (A)"=w454, "start"=w450, "compliance (V)"=w452, "total points"=w453, "step"=w448, "Mode"=w458) -> ("total points 2"=w451:u16, "compliance"=w449:dbl)  [unwired: 1 in, 1 out]
                      n175 = call "HP415xA _Config-Sweep-Secondary Sour.vi"("compliance"=w449, "step"=w448, "error in (no error)"=w456, "total points"=w451, "start"=w450, "VISA session"=w457) -> ("error out"=w455:errorcluster)  [unwired: 1 in]
                      n176 = local write "error?"(w455) -> ()
                    }
                  }
                }
                frame True {
                  n177 = local read "Mode"() -> (w466:u16)
                  n178 = call "compliancevi3subvi.vi"("compliance (A)"=w464, "start"=w459, "compliance (V)"=w463, "total points"=w465, "step"=w461, "Mode"=w466) -> ("total points 2"=w460:u16, "compliance"=w462:dbl)  [unwired: 1 in, 1 out]
                  n179 = call "HP415xA _Config-Sweep-Secondary Sour.vi"("compliance"=w462, "step"=w461, "error in (no error)"=w468, "total points"=w460, "start"=w459, "VISA session"=w469) -> ("error out"=w467:errorcluster)  [unwired: 1 in]
                  n180 = local write "error?"(w467) -> ()
                }
              }
            }
          }
        }
        frame True {
          w478 = u16 2 items=["disabled", "Var1", "Var2", "Var1'", "Constant"] ("Function 2")
          n181 = local read "error?"() -> (w480:errorcluster)
          n182 = local read "Mode"() -> (w488:u16)
          n183 = local read "Function 2"() -> (w479:u16)
          n184 = call "compliancesubvi2.vi"("compliance (V)"=w487, "Mode"=w488, "compliance (A)"=w486) -> ("compliance"=w489:dbl)  [unwired: 3 in, 1 out]
          n185 = call "HP415xA _Config-Sweep-Primary Sour.vi"("step (linear only)"=w483, "stop"=w482, "start"=w481, "compliance"=w489, "error in (no error)"=w480, "sweep mode"=w484, "sweep spacing (linear: 0)"=w485, "VISA session"=w470) -> ("error out"=w471:errorcluster)  [unwired: 2 in]
          n186 = Equal?(x=w479, y=w478) -> (x = y?=w477:bool)
          n187 = case shown="True" w477 {
            tunnel: w476 -> [w495 w539]
            tunnel: w475 -> [w496 w538]
            tunnel: w474 -> [w493 w535]
            tunnel: w473 -> [w494 w537]
            tunnel: w472 -> [w492 w533]
            tunnel: w471 -> [w491 w542]
            tunnel: w470 -> [w490 w540]
            frame False {
              w499 = u16 2 items=["disabled", "Var1", "Var2", "Var1'", "Constant"] ("Function 2")
              n188 = local read "Function 3"() -> (w498:u16)
              n189 = Equal?(x=w498, y=w499) -> (x = y?=w497:bool)
              n190 = case shown="True" w497 {
                tunnel: w496 -> [w504 w522]
                tunnel: w495 -> [w505 w523]
                tunnel: w494 -> [w502 w528]
                tunnel: w493 -> [w503 w525]
                tunnel: w492 -> [w501 w524]
                tunnel: w491 -> [w506 w531]
                tunnel: w490 -> [w500 w529]
                frame False {
                  w509 = u16 2 items=["disabled", "Var1", "Var2", "Var1'", "Constant"] ("Function 2")
                  n191 = local read "Function 4"() -> (w508:u16)
                  n192 = Equal?(x=w508, y=w509) -> (x = y?=w507:bool)
                  n193 = case shown="True" w507 {
                    tunnel: w506 -> [w510 w521]
                    tunnel: w505 -> [_ w511]
                    tunnel: w504 -> [_ w512]
                    tunnel: w503 -> [_ w513]
                    tunnel: w502 -> [_ w518]
                    tunnel: w501 -> [_ w515]
                    tunnel: w500 -> [_ w519]
                    frame False {
                      n194 = local write "error?"(w510) -> ()
                    }
                    frame True {
                      n195 = local read "Mode 4"() -> (w517:u16)
                      n196 = call "compliancevi3subvi.vi"("compliance (A)"=w511, "start"=w513, "compliance (V)"=w512, "total points"=w518, "step"=w515, "Mode"=w517) -> ("total points 2"=w514:u16, "compliance"=w516:dbl)  [unwired: 1 in, 1 out]
                      n197 = call "HP415xA _Config-Sweep-Secondary Sour.vi"("compliance"=w516, "step"=w515, "error in (no error)"=w521, "total points"=w514, "start"=w513, "VISA session"=w519) -> ("error out"=w520:errorcluster)  [unwired: 1 in]
                      n198 = local write "error?"(w520) -> ()
                    }
                  }
                }
                frame True {
                  n199 = local read "Mode 3"() -> (w532:u16)
                  n200 = call "compliancevi3subvi.vi"("compliance (A)"=w523, "start"=w525, "compliance (V)"=w522, "total points"=w528, "step"=w524, "Mode"=w532) -> ("total points 2"=w527:u16, "compliance"=w526:dbl)  [unwired: 1 in, 1 out]
                  n201 = call "HP415xA _Config-Sweep-Secondary Sour.vi"("compliance"=w526, "step"=w524, "error in (no error)"=w531, "total points"=w527, "start"=w525, "VISA session"=w529) -> ("error out"=w530:errorcluster)  [unwired: 1 in]
                  n202 = local write "error?"(w530) -> ()
                }
              }
            }
            frame True {
              n203 = local read "Mode 2"() -> (w543:u16)
              n204 = call "compliancevi3subvi.vi"("compliance (A)"=w539, "start"=w535, "compliance (V)"=w538, "total points"=w537, "step"=w533, "Mode"=w543) -> ("total points 2"=w536:u16, "compliance"=w534:dbl)  [unwired: 1 in, 1 out]
              n205 = call "HP415xA _Config-Sweep-Secondary Sour.vi"("compliance"=w534, "step"=w533, "error in (no error)"=w542, "total points"=w536, "start"=w535, "VISA session"=w540) -> ("error out"=w541:errorcluster)  [unwired: 1 in]
              n206 = local write "error?"(w541) -> ()
            }
          }
        }
      }
    }
    frame #4 {
      # "This step sets the integration time."
      n207 = local read "VISA session"() -> (w544:refnum<visa-resource-name>)
      n208 = local read "error?"() -> (w548:errorcluster)
      n209 = call "HP415xA _Config-Meas-Timing.vi"("error in (no error)"=w548, "wait time parameter"="wait time parameter", "integration time"="integration time", "VISA session"=w544) -> ("error out"=w547:errorcluster)  [unwired: 2 in]
      n210 = local write "error?"(w547) -> ()
    }
    frame #5 {
      w584 = u32 1 items=["stop  ", "single  ", "single-append  ", "stress start  ", "continuous  ", "standby on  ", "standby off  ", "zero  "] ("function (stop:0)")
      w588 = u16 2 items=["disabled", "Var1", "Var2", "Var1'", "Constant"] ("Function")
      w593 = u16 1 items=["disabled", "Var1", "Var2", "Var1'", "Constant"] ("Function")
      n211 = local read "Function"() -> (w595:u16)
      n212 = local read "Function"() -> (w587:u16)
      n213 = Equal?(x=w595, y=w593) -> (x = y?=w594:bool)
      n214 = Equal?(x=w587, y=w588) -> (x = y?=w586:bool)
      n215 = case shown="False" w594 {
        tunnel: [w958 w973] -> w589
        tunnel: [w959 w972] -> _
        tunnel: w593 -> [w956 _]
        frame False {
          n216 = local read "Function 2"() -> (w960:u16)
          n217 = Equal?(x=w960, y=w956) -> (x = y?=w957:bool)
          n218 = case shown="False" w957 {
            tunnel: [w961 w971] -> w959
            tunnel: [w962 w970] -> w958
            tunnel: w956 -> [w965 _]
            frame False {
              n219 = local read "Function 3"() -> (w964:u16)
              n220 = Equal?(x=w964, y=w965) -> (x = y?=w963:bool)
              n221 = case shown="True" w963 {
                tunnel: [w967 w969] -> w962
                tunnel: [w966 w968] -> w961
                frame False {
                  n222 = local read "Vname 4"() -> (w967:string)
                  n223 = local read "Iname 4"() -> (w966:string)
                }
                frame True {
                  n224 = local read "Vname 3"() -> (w969:string)
                  n225 = local read "Iname 3"() -> (w968:string)
                }
              }
            }
            frame True {
              n226 = local read "Vname 2"() -> (w970:string)
              n227 = local read "Iname 2"() -> (w971:string)
            }
          }
        }
        frame True {
          n228 = local read "Vname"() -> (w973:string)
          n229 = local read "Iname"() -> (w972:string)
        }
      }
      n230 = case shown="False" w586 {
        tunnel: [w900 w953] -> w559
        tunnel: [w899 TRUE ("x = y?")] -> w565
        frame False {
          w903 = u16 2 items=["disabled", "Var1", "Var2", "Var1'", "Constant"] ("Function")
          n231 = local read "Function 2"() -> (w902:u16)
          n232 = Equal?(x=w902, y=w903) -> (x = y?=w901:bool)
          n233 = case shown="False" w901 {
            tunnel: [w905 w943] -> w900
            tunnel: [w904 TRUE ("x = y?")] -> w899
            frame False {
              w908 = u16 2 items=["disabled", "Var1", "Var2", "Var1'", "Constant"] ("Function")
              n234 = local read "Function 3"() -> (w907:u16)
              n235 = Equal?(x=w907, y=w908) -> (x = y?=w906:bool)
              n236 = case shown="False" w906 {
                tunnel: [w913 w933] -> w905
                tunnel: [w909 TRUE ("x = y?")] -> w904
                frame False {
                  w912 = u16 2 items=["disabled", "Var1", "Var2", "Var1'", "Constant"] ("Function")
                  n237 = local read "Function 4"() -> (w911:u16)
                  n238 = Equal?(x=w911, y=w912) -> (x = y?=w910:bool)
                  n239 = case shown="False" w910 {
                    tunnel: ["0" ("Vname 4") w923] -> w913
                    tunnel: [FALSE ("x = y?") TRUE ("x = y?")] -> w909
                    frame False {
                    }
                    frame True {
                      w917 = u16 2 items=["V", "I", "VPulse", "IPulse", "Common"] ("Mode 2")
                      w920 = u16 0 items=["V", "I", "VPulse", "IPulse", "Common"] ("Mode 2")
                      n240 = local read "Mode 4"() -> (w919:u16)
                      n241 = Equal?(x=w920, y=w919) -> (x = y?=w921:bool)
                      n242 = Equal?(x=w919, y=w917) -> (x = y?=w918:bool)
                      n243 = Or(x=w921, y=w918) -> (x .or. y?=w916:bool)
                      n244 = case shown="False" w916 {
                        tunnel: [w924 w925] -> w923
                        frame False {
                          n245 = local read "Iname 4"() -> (w924:string)
                        }
                        frame True {
                          n246 = local read "Vname 4"() -> (w925:string)
                        }
                      }
                    }
                  }
                }
                frame True {
                  w929 = u16 2 items=["V", "I", "VPulse", "IPulse", "Common"] ("Mode 2")
                  w928 = u16 0 items=["V", "I", "VPulse", "IPulse", "Common"] ("Mode 2")
                  n247 = local read "Mode 3"() -> (w927:u16)
                  n248 = Equal?(x=w928, y=w927) -> (x = y?=w931:bool)
                  n249 = Equal?(x=w927, y=w929) -> (x = y?=w930:bool)
                  n250 = Or(x=w931, y=w930) -> (x .or. y?=w926:bool)
                  n251 = case shown="False" w926 {
                    tunnel: [w934 w935] -> w933
                    frame False {
                      n252 = local read "Iname 3"() -> (w934:string)
                    }
                    frame True {
                      n253 = local read "Vname 3"() -> (w935:string)
                    }
                  }
                }
              }
            }
            frame True {
              w937 = u16 2 items=["V", "I", "VPulse", "IPulse", "Common"] ("Mode 2")
              w938 = u16 0 items=["V", "I", "VPulse", "IPulse", "Common"] ("Mode 2")
              n254 = local read "Mode 2"() -> (w939:u16)
              n255 = Equal?(x=w938, y=w939) -> (x = y?=w941:bool)
              n256 = Equal?(x=w939, y=w937) -> (x = y?=w940:bool)
              n257 = Or(x=w941, y=w940) -> (x .or. y?=w936:bool)
              n258 = case shown="True" w936 {
                tunnel: [w944 w945] -> w943
                frame False {
                  n259 = local read "Iname 2"() -> (w944:string)
                }
                frame True {
                  n260 = local read "Vname 2"() -> (w945:string)
                }
              }
            }
          }
        }
        frame True {
          w950 = u16 2 items=["V", "I", "VPulse", "IPulse", "Common"] ("Mode")
          w951 = u16 0 items=["V", "I", "VPulse", "IPulse", "Common"] ("Mode")
          n261 = local read "Mode"() -> (w949:u16)
          n262 = Equal?(x=w949, y=w951) -> (x = y?=w948:bool)
          n263 = Equal?(x=w949, y=w950) -> (x = y?=w947:bool)
          n264 = Or(x=w948, y=w947) -> (x .or. y?=w946:bool)
          n265 = case shown="True" w946 {
            tunnel: [w954 w955] -> w953
            frame False {
              n266 = local read "Iname"() -> (w954:string)
            }
            frame True {
              n267 = local read "Vname"() -> (w955:string)
            }
          }
        }
      }
      n268 = local read "error?"() -> (w576:errorcluster)
      n269 = Unbundle("Y2 axis settings") -> ("Y2 axis on/off"=w568:bool, "MINIMUM"=w581:ext, "MAXIMUM"=w580:ext, "Variable name"=w572:string, "LIN or LOG axis"=w579:string)
      n270 = local read "Var2 step settings"() -> (w591:T3)
      n271 = local read "Var1 sweep settings"() -> (w592:T4)
      n272 = local read "VISA session"() -> (w560:refnum<visa-resource-name>)
      n273 = call "Y1subvi.vi"("MAXIMUM"="MAXIMUM", "Variable name"="Y1 axis", "error in (no error)"=w576, "MINIMUM"="MINIMUM", "LIN or LOG axis"="LIN", "VISA resource name"=w560) -> ("error out"=w577:errorcluster)
      n274 = case shown="False" w568 {
        tunnel: w577 -> [w891 w898]
        tunnel: w560 -> [_ w897]
        tunnel: w581 -> [_ w896]
        tunnel: w580 -> [_ w895]
        tunnel: w572 -> [_ w894]
        tunnel: w579 -> [_ w893]
        tunnel: [w891 w892] -> w578
        frame False {
        }
        frame True {
          n275 = call "Y2subvi.vi"("MAXIMUM"=w895, "Variable name"=w894, "error in (no error)"=w898, "MINIMUM"=w896, "LIN or LOG axis"=w893, "VISA resource name"=w897) -> ("error out"=w892:errorcluster)
        }
      }
      n276 = Unbundle(w591) -> ("total points"=w590:u16)  [unwired: 4 out]
      n277 = Decrement(x=w590) -> (x-1=w550:u16)
      n278 = Unbundle(w592) -> ("start"=w558:dbl)  [unwired: 6 out]
      n279 = call "HP415xA Op-Start-Stop.vi"("error in (no error)"=w578, "function (stop:0)"=w584, "wait until finish"=TRUE, "VISA session"=w560) -> ("error out"=w583:errorcluster)  [unwired: 6 in, 1 out]
      n280 = call "HP415xA Op-Download Trace.vi"("error in (no error)"=w583, "trace (variable) name"=w589, "VISA session"=w560) -> ("error out"=w598:errorcluster, "trace"=w566:dbl[])
      n281 = call "HP415xA Op-Download Trace.vi"("error in (no error)"=w598, "trace (variable) name"="Y1 axis", "VISA session"=w560) -> ("error out"=w573:errorcluster, "trace"=w561:dbl[])
      n282 = case shown="False" w568 {
        tunnel: w573 -> [w876 w884]
        tunnel: w560 -> [_ w883]
        tunnel: w572 -> [_ w882]
        tunnel: [w876 w881] -> w562
        tunnel: w566 -> [w874 w880]
        tunnel: w561 -> [w875 w879]
        tunnel: [w873 w878] -> w569
        tunnel: [dbl[] [] ("trace") w877] -> w567
        frame False {
          n283 = Bundle("trace"=w874, "trace"=w875) -> (w873:cluster{"trace":dbl[], "trace":dbl[]})  [unwired: 1 in]
        }
        frame True {
          n284 = call "HP415xA Op-Download Trace.vi"("error in (no error)"=w884, "trace (variable) name"=w882, "VISA session"=w883) -> ("error out"=w881:errorcluster, "trace"=w877:dbl[])
          n285 = stacked-sequence {
            tunnel: w877 -> [_ w889]
            tunnel: w880 -> [w887 w888]
            tunnel: w879 -> [w886 _]
            tunnel: [w885 _] -> w878
            frame #0 {
              n286 = Bundle("trace"=w887, "trace"=w886) -> (w885:cluster{"trace":dbl[], "trace":dbl[]})  [unwired: 1 in]
            }
            frame #1 {
              n287 = Bundle("trace"=w888, "trace"=w889) -> (→"graphic display 2":cluster{"trace":dbl[], "trace":dbl[]})  [unwired: 1 in]
            }
          }
        }
      }
      "graphic display" <- w569
      n288 = case shown="True" w565 {
        tunnel: w558 -> [_ w744]
        tunnel: w561 -> [w603 w743]
        tunnel: w566 -> [w604 w741]
        tunnel: w550 -> [_ w740]
        tunnel: w560 -> [_ w736]
        tunnel: w562 -> [_ w735]
        tunnel: [w605 w734] -> w564
        tunnel: w559 -> [_ w733]
        tunnel: w559 -> [_ w726]
        tunnel: [dbl[] [] ("trace") w732] -> w563
        tunnel: w557 -> [_ w729]
        tunnel: w556 -> [_ w728]
        tunnel: w555 -> [_ w677]
        tunnel: [_ w653] -> w554
        tunnel: [_ w655] -> w553
        tunnel: w552 -> [_ w694]
        tunnel: w551 -> [_ w693]
        tunnel: w550 -> [_ _]
        tunnel: w549 -> [_ w688]
        frame False {
          n289 = Build Array(w604, w603) -> (w600:dbl[][])
          n290 = local read "error? 2"() -> (w605:errorcluster)
          n291 = call-poly <vilib>:"Write To Spreadsheet File.vi"("transpose? (no:F)"=TRUE ("append to file? (new file:F)"), "format (%.3f)"="%.5e", "2D data"=w600) -> ()  [unwired: 5 in, 1 out]
        }
        frame True {
          w647 = 2
          w648 = 2
          w661 = 0
          w659 = 0
          (unwired) 0.000115
          w718 = "%s"
          w668 = "\r"
          n292 = Initialize Array("") -> (w707:string[])  [unwired: 1 in]
          n293 = call "HP415xA Op-Download Trace.vi"("error in (no error)"=w735, "trace (variable) name"=w733, "VISA session"=w736) -> ("error out"=w734:errorcluster, "trace"=w732:dbl[])
          n294 = for {
            N: w740 -> [w799]
            shift-right: [w816] -> w653
            shift-left: w741 -> [w812]
            tunnel: w744 -> [w818]
            tunnel: [w817] -> _ mode=indexing
            shift-right: [w813] -> w655
            shift-left: w743 -> [w815]
            tunnel: [w814] -> w742 mode=indexing
            shift-right: [w809] -> w722
            shift-left: w732 -> [w811]
            tunnel: w726 -> [_]
            tunnel: [w803] -> w724 mode=indexing
            shift-right: [w802] -> w711
            shift-left: w707 -> [w801]
            tunnel: [w799] -> _ mode=indexing
            n295 = Search 1D Array(1D array=w812, element=w818, start index (0)=1) -> (index of element=w810:i32)
            n296 = Split 1D Array(array=w811, index=w810) -> (first subarray=w807:dbl[], second subarray=w809:dbl[])
            n297 = Array Size(array=w807) -> (size(s)=w806:i32)
            n298 = Decrement(x=w806) -> (x-1=w805:i32)
            n299 = Split 1D Array(array=w815, index=w810) -> (first subarray=w814:dbl[], second subarray=w813:dbl[])
            n300 = Split 1D Array(array=w812, index=w810) -> (first subarray=w817:dbl[], second subarray=w816:dbl[])
            n301 = Array Subset(array=w807, index=w805) -> (w808:dbl[])  [unwired: 1 in]
            n302 = Number To Exponential String(number=w808) -> (E-format string=w804:string[])  [unwired: 3 in]
            n303 = Concatenate Strings(w804) -> (w803:string)
            n304 = Build Array (concatenate)("Id", w801) -> (w802:string[])
          }
          n305 = Build Array (concatenate)(w653, w742, w655) -> (w739:dbl[][])
          n306 = Transpose 2D Array(2D array=w739) -> (transposed array=w737:dbl[][])
          n307 = Array To Spreadsheet String(array=w737, 3:"%.5e" ("format string")) -> (spreadsheet string=w727:string)  [unwired: 1 in]
          n308 = local read "Temp (K)"() -> (w607:dbl)
          n309 = Format Value(format string="%#g", value (0)=w607) -> (output string=w644:string)  [unwired: 1 in]
          n310 = Build Array("Sample Temp (K):", w644) -> (w643:string[])
          n311 = Build Array("Vg", "Id") -> (w712:string[])
          n312 = Array Size(array=w722) -> (size(s)=w723:i32)
          n313 = Reshape Array(w643, 1 ("start index (0)")) -> (w640:string[])
          n314 = Decrement(x=w723) -> (x-1=w721:i32)
          n315 = Array Subset(array=w722, index=w721) -> (w720:dbl[])  [unwired: 1 in]
          n316 = Insert Into Array(array=w712, index=2, new element=w711) -> (w710:string[])
          n317 = Number To Exponential String(number=w720) -> (E-format string=w716:string[])  [unwired: 3 in]
          n318 = Array To Spreadsheet String(array=w640, 3:"%s") -> (spreadsheet string=w639:string)  [unwired: 1 in]
          n319 = Array To Spreadsheet String(array=w710, 3:w718) -> (spreadsheet string=w717:string)  [unwired: 1 in]
          n320 = Concatenate Strings(w716) -> (w715:string)
          n321 = Build Array (concatenate)("Vd=", w724, w715) -> (w719:string[])
          n322 = Array To Spreadsheet String(array=w719, 3:w718) -> (spreadsheet string=w725:string)  [unwired: 1 in]
          n323 = Fract/Exp String To Number(string="") -> (number=w628:dbl)  [unwired: 3 in, 1 out]
          n324 = local read "Vt"() -> (w638:dbl)
          n325 = Build Array("Mobility-Sat (cm^2/Vs):", "Mobility-Lin (cm^2/Vs):", "On/Off I-Sat:", "Off I-Sat (A):", "Vt-Sat (V):", "STS-Sat (V/decade):", "Trap Density-VT (Traps/Vcm^2):", "Trap Density-STS (Traps/Vcm^2):") -> (w675:string[])
          n326 = Array Size(array=w653) -> (size(s)=w681:i32)
          n327 = Subtract(x=w681, y="NumPts") -> (x-y=w692:dbl)
          n328 = Initialize Array(0) -> (w691:i32[])  [unwired: 1 in]
          n329 = Initialize Array(w659, w648) -> (w660:i32[])
          n330 = Initialize Array(w659, w648) -> (w658:i32[])
          n331 = Initialize Array(w659) -> (w663:i32[])  [unwired: 1 in]
          n332 = for {
            N: w681 -> [w747]
            shift-right: [w750] -> w680
            shift-left: w655 -> [w751]
            i -> [w746]
            n333 = Subtract(x=w747, y=w746) -> (x-y=w745:i32)
            n334 = Index Array(array=w751, index=w745) -> (element=w748:dbl)
            n335 = Greater Or Equal To 0?(x=w748) -> (x >= 0?=w749:bool)
            n336 = case shown="False" w749 {
              tunnel: w751 -> [w752 w755]
              tunnel: w745 -> [_ w753]
              tunnel: [w752 w754] -> w750
              frame False {
              }
              frame True {
                n337 = Delete From Array(array=w755, index=w753) -> (array with subset deleted=w754:dbl[])  [unwired: 1 in, 1 out]
              }
            }
          }
          n338 = for {
            N: w692 -> [_]
            shift-right: [w793] -> _
            shift-left: w653 -> [w793]
            shift-right: [w794] -> _
            shift-left: w655 -> [w794]
            shift-right: [w798] -> w697
            shift-left: w691 -> [w797]
            shift-right: [w796] -> w695
            shift-left: w663 -> [w795]
            tunnel: "NumPts" -> [w788]
            shift-right: [w784] -> w662
            shift-left: w660 -> [w787]
            shift-right: [w781] -> w651
            shift-left: w658 -> [w782]
            i -> [w785]
            n339 = Array Subset(array=w793, index=w785, length=w788) -> (w783:dbl[])
            n340 = Array Subset(array=w794, index=w785, length=w788) -> (w792:dbl[])
            n341 = Absolute Value(x=w792) -> (abs(x)=w791:dbl[])
            n342 = Build Array (concatenate)(w782, w783) -> (w781:dbl[])
            n343 = Square Root(x=w791) -> (sqrt(x)=w786:dbl[])
            n344 = call <vilib>:"Linear Fit.vi"("Y"=w786, "X"=w783) -> ("Best Linear Fit"=w790:dbl[], "slope"=w780:dbl, "intercept"=w778:dbl)  [unwired: 9 in, 2 out]
            n345 = Insert Into Array(array=w787, index=w785, new element=w786) -> (w784:i32[])
            n346 = call <vilib>:"Goodness of Fit.vi"("Best Fit"=w790, "Y"=w786) -> ("R-square"=w789:dbl)  [unwired: 6 in, 3 out]
            n347 = Negate(x=w780) -> (-x=w779:dbl)
            n348 = Divide(x=w779, y=w778) -> ()  [unwired: 1 out]
            n349 = Build Array (concatenate)(w795, w789) -> (w796:dbl[])
            n350 = Build Array (concatenate)(w797, w780) -> (w798:dbl[])
          }
          n351 = Absolute Value(x=w655) -> (abs(x)=w657:dbl[])
          n352 = Array Max & Min(array=w680) -> (max value=w678:dbl, min value=w679:dbl)  [unwired: 2 out]
          n353 = Square Root(x=w657) -> (sqrt(x)=w656:dbl[])
          n354 = Initialize Array(w661, w647) -> (w650:i32[])
          n355 = Initialize Array(w661, w647) -> (w667:i32[])
          n356 = Divide(x=w679, y=w678) -> (x/y=w630:dbl)
          n357 = for {
            N: 20 -> [_]
            shift-right: [w776] -> _
            shift-left: w695 -> [w777]
            shift-right: [w768] -> _
            shift-left: w697 -> [w766]
            shift-right: [w767] -> w698
            shift-left: w667 -> [w775]
            shift-right: [w774] -> w689
            shift-left: w667 -> [w773]
            shift-right: [w764] -> _
            shift-left: w662 -> [w765]
            shift-right: [w763] -> w617
            shift-left: w650 -> [w771]
            shift-right: [w756] -> _
            shift-left: w651 -> [w758]
            shift-right: [w760] -> w616
            shift-left: w650 -> [w759]
            w762 = 1
            n358 = Array Max & Min(array=w777) -> (max value=w772:dbl, max index (indices)=w757:i32)  [unwired: 2 out]
            n359 = Array Subset(array=w758, index=w757, length=w762) -> (w761:dbl[])
            n360 = Array Subset(array=w765, index=w757, length=w762) -> (w770:i32[])
            n361 = Array Subset(array=w766, index=w757, length=w762) -> (w769:dbl[])
            n362 = Build Array (concatenate)(w775, w769) -> (w767:dbl[])
            n363 = Delete From Array(array=w777, index=w757) -> (array with subset deleted=w776:dbl[])  [unwired: 1 in, 1 out]
            n364 = Build Array (concatenate)(w759, w761) -> (w760:dbl[])
            n365 = Build Array (concatenate)(w773, w772) -> (w774:dbl[])
            n366 = Build Array (concatenate)(w771, w770) -> (w763:i32[])
            n367 = Delete From Array(array=w765, index=w757) -> (array with subset deleted=w764:i32[])  [unwired: 1 in, 1 out]
            n368 = Delete From Array(array=w758, index=w757) -> (array with subset deleted=w756:dbl[])  [unwired: 1 in, 1 out]
            n369 = Delete From Array(array=w766, index=w757) -> (array with subset deleted=w768:dbl[])  [unwired: 1 in, 1 out]
          }
          "Max R" <- w689
          n370 = local write "On/Off Current"(w630) -> ()
          n371 = Bundle("trace"=w653, w656) -> (w654:cluster{"trace":dbl[], dbl[]})  [unwired: 1 in]
          n372 = Fract/Exp String To Number(string=w694) -> (number=w665:dbl)  [unwired: 3 in, 1 out]
          n373 = local read "Vt"() -> (w637:dbl)
          n374 = Fract/Exp String To Number(string=w693) -> (number=w666:dbl)  [unwired: 3 in, 1 out]
          n375 = Fract/Exp String To Number(string=w688) -> (number=w683:dbl)  [unwired: 3 in, 1 out]
          n376 = Array Max & Min(array=w698) -> (min value=w649:dbl, min index (indices)=w619:i32)  [unwired: 2 out]
          n377 = Multiply(x=w619, y="NumPts") -> (x*y=w621:dbl)
          n378 = Array Subset(array=w616, index=w621, length="NumPts") -> (w622:dbl[])
          n379 = Array Subset(array=w617, index=w621, length="NumPts") -> (w623:i32[])
          n380 = call <vilib>:"Linear Fit.vi"("Y"=w623, "X"=w622) -> ("slope"=w626:dbl, "intercept"=w624:dbl)  [unwired: 9 in, 3 out]
          n381 = Negate(x=w624) -> (-x=w625:dbl)
          n382 = Divide(x=w625, y=w626) -> (x/y=w620:dbl)
          n383 = Bundle(w622, w623) -> (w615:cluster{dbl[], i32[]})  [unwired: 1 in]
          n384 = local write "Vt"(w620) -> ()
          n385 = Build Array(w654, w615) -> (→"XY Graph":cluster{"trace":dbl[], dbl[]}[])
          n386 = Absolute Value(x=w637) -> (abs(x)=w636:dbl)
          n387 = Square(x=w649) -> (x^2=w699:dbl)
          n388 = Multiply(x=2, y=w699) -> (x*y=w700:dbl)
          n389 = Multiply(x=3.9, y=8.854e-12) -> (x*y=w685:dbl)
          n390 = Multiply(x=w666, y=w700) -> (x*y=w701:dbl)
          n391 = Multiply(x=w683, y=1e-09) -> (x*y=w682:dbl)
          n392 = Divide(x=w685, y=w682) -> (x/y=w635:dbl)
          n393 = Multiply(x=w636, y=w635) -> (x*y=w634:dbl)
          n394 = Divide(x=w634, y=1.602e-19) -> (x/y=w631:dbl)
          n395 = Multiply(x=w665, y=w635) -> (x*y=w702:dbl)
          n396 = Divide(x=w701, y=w702) -> (x/y=w704:dbl)
          n397 = Multiply(x=w704, y=10000) -> (x*y=w632:dbl)
          n398 = Build Array(w632, w630, w638, w628, w631, w628) -> (w674:dbl[])
          n399 = Number To Exponential String(number=w674) -> (E-format string=w673:string[])  [unwired: 3 in]
          n400 = Build Array(w675, w673) -> (w672:string[][])
          n401 = Transpose 2D Array(2D array=w672) -> (transposed array=w671:string[][])
          n402 = Array To Spreadsheet String(array=w671, 3:"%s") -> (spreadsheet string=w669:string)  [unwired: 1 in]
          n403 = Concatenate Strings(w729, w668, w728, w668, w677, w639, w668, w669, w668, w725, w717, w727, "\r") -> (w731:string)
          n404 = call <vilib>:"Write Characters To File.vi"("append to file? (new file:F)"=TRUE, "character string"=w731, "file path (dialog if empty)"="Input Path") -> ("new file path (Not A Path if cancelled)"=w627:path)  [unwired: 2 in]
          n405 = local write "Output Path"(w627) -> ()
          n406 = local write "Trap Density-VT"(w631) -> ()
          n407 = local write "Mobility"(w632) -> ()
        }
      }
      n408 = case shown="True" w568 {
        tunnel: w550 -> [_ w825]
        tunnel: w565 -> [_ w826]
        tunnel: w566 -> [_ w824]
        tunnel: w558 -> [_ w823]
        tunnel: w567 -> [_ w822]
        tunnel: w563 -> [_ w821]
        tunnel: w559 -> [_ w820]
        frame False {
        }
        frame True {
          n409 = case shown="True" w826 {
            tunnel: w825 -> [_ w842]
            tunnel: w824 -> [w830 w857]
            tunnel: w823 -> [_ w856]
            tunnel: w822 -> [w831 w855]
            tunnel: w821 -> [_ w854]
            tunnel: w820 -> [_ w837]
            frame False {
              n410 = Build Array(w830, w831) -> (w829:dbl[][])
              n411 = call-poly <vilib>:"Write To Spreadsheet File.vi"("transpose? (no:F)"=TRUE, "format (%.3f)"="%.5e", "2D data"=w829) -> ()  [unwired: 5 in, 1 out]
            }
            frame True {
              n412 = for {
                N: w842 -> [_]
                shift-right: [w868] -> w853
                shift-left: w857 -> [w869]
                tunnel: w856 -> [w871]
                tunnel: [w867] -> _ mode=indexing
                shift-right: [w864] -> w851
                shift-left: w855 -> [w866]
                tunnel: [w865] -> w852 mode=indexing
                shift-right: [w861] -> w846
                shift-left: w854 -> [w862]
                tunnel: [w858] -> w843 mode=indexing
                n413 = Search 1D Array(1D array=w869, element=w871, start index (0)=1) -> (index of element=w863:i32)
                n414 = Split 1D Array(array=w869, index=w863) -> (first subarray=w867:dbl[], second subarray=w868:dbl[])
                n415 = Split 1D Array(array=w866, index=w863) -> (first subarray=w865:dbl[], second subarray=w864:dbl[])
                n416 = Split 1D Array(array=w862, index=w863) -> (first subarray=w859:dbl[], second subarray=w861:dbl[])
                n417 = Index Array(array=w859, index=1) -> (element=w858:dbl)
              }
              n418 = Build Array (concatenate)(w853, w852, w851) -> (w850:dbl[][])
              n419 = Index Array(array=w846, index=1) -> (element=w844:dbl)
              n420 = Transpose 2D Array(2D array=w850) -> (transposed array=w849:dbl[][])
              n421 = Insert Into Array(array=w843, index=w842, new element=w844) -> (w841:dbl[])
              n422 = Array To Spreadsheet String(delimiter (Tab)=",", array=w841, 3:"%.5e" ("format string")) -> (spreadsheet string=w835:string)
              n423 = Array To Spreadsheet String(delimiter (Tab)=",", array=w849, 3:"%.5e" ("format string")) -> (spreadsheet string=w833:string)
              n424 = Concatenate Strings(w837, "," ("string")) -> (w836:string)
              n425 = Concatenate Strings(w836, w835) -> (w834:string)
              n426 = Concatenate Strings(w834, w833) -> (w832:string)
              n427 = call <vilib>:"Write Characters To File.vi"("character string"=w832) -> ()  [unwired: 4 in, 1 out]
            }
          }
        }
      }
      n428 = call "HP415xA Sys-Error Query.vi"("VISA session"=w560, "error in (no error)"=w564) -> ("error out"=w596:errorcluster)  [unwired: 2 in, 1 out]
      n429 = call "HP415xA  Close.vi"("error in (no error)"=w596, "VISA session"=w560) -> ("error out"=w597:errorcluster)
      n430 = local write "error?"(w597) -> ()
    }
    frame #6 {
      n431 = flat-sequence {
        frame #0 {
          n432 = local read "Output Path"() -> (w988:path)
          n433 = local read "Sample Properties:"() -> (w984:T1)
          n434 = local read "Temp (K)"() -> (w975:dbl)
          n435 = call "sub_thresh_swing_subvi.vi"("Path"=w988) -> ("Sub Threshold Swing"=w974:dbl)  [unwired: 10 in, 4 out]
          n436 = Unbundle By Name(w984) -> ("SiO2 Thickness"=w977:string)
          n437 = Equal To 0?(x=w975) -> (x = 0?=w987:bool)
          n438 = local write "STS"(w974) -> ()
          n439 = case shown="True" w987 {
            tunnel: [w989 290] -> w986
            tunnel: w975 -> [w989 _]
            frame False {
            }
            frame True {
            }
          }
          n440 = Fract/Exp String To Number(string=w977) -> (number=w979:dbl)  [unwired: 3 in, 1 out]
          n441 = Multiply(x=3.9, y=8.854e-12) -> (x*y=w983:dbl)
          n442 = Multiply(x=w979, y=1e-09) -> (x*y=w980:dbl)
          n443 = Divide(x=w983, y=w980) -> (x/y=w976:dbl)
          n444 = call "Trap Density_STS.vi"("Temp (T) [K]"=w986, "S.T.S. (S)"=w974, "Dielectric"=w976) -> ("Trap Density (N)"=w985:dbl)  [unwired: 8 in]
          n445 = local write "Trap Density-STS"(w985) -> ()
        }
        frame #1 {
          n446 = local read "Output Path"() -> (w991:path)
          n447 = call-poly <vilib>:"Read From Spreadsheet File.vi"("file path (dialog if empty)"=w991) -> ("all rows"=w998:string[][])  [unwired: 6 in, 4 out]
          n448 = Array Subset(array=w998, index (col)=0, length (col)=1) -> (w1006:string[][])  [unwired: 2 in]
          n449 = Reshape Array(w1006, 100) -> (w1003:string[])
          n450 = Search 1D Array(1D array=w1003, element="S.T.S. (V/decade):") -> (index of element=w1001:i32)  [unwired: 1 in]
          n451 = Search 1D Array(1D array=w1003, element="Trap Density-STS (Traps/Vcm^2):") -> (index of element=w995:i32)  [unwired: 1 in]
          n452 = local read "Trap Density-STS"() -> (w994:dbl)
          n453 = local read "STS"() -> (w1002:dbl)
          n454 = Number To Exponential String(number=w1002) -> (E-format string=w999:string)  [unwired: 3 in]
          n455 = Replace Array Subset(array=w998, new element=w999, index (row)=w1001, index (col)=1) -> (w997:string[][])
          n456 = Number To Exponential String(number=w994) -> (E-format string=w993:string)  [unwired: 3 in]
          n457 = Replace Array Subset(array=w997, new element=w993, index (row)=w995, index (col)=1) -> (w992:string[][])
          "Array" <- w992
          n458 = call-poly <vilib>:"Write To Spreadsheet File.vi"("2D data"=w992, "file path (dialog if empty)"=w991) -> ()  [unwired: 6 in, 1 out]
        }
      }
    }
  }
